vi "Main.vi"() -> ()   [LabVIEW 2020]
doc: "Use this template to build a simple state machine design pattern. Each state executes code and determines which state to transition to."
uses:
  Type Definitions/Data.ctl
  Type Definitions/Error Levels.ctl
  <userlib>/RxnRover/DynamicReentrant/Dynamic Reentrant.lvlib
  <userlib>/RxnRover/DynamicReentrant/src/Type Defs/Message.ctl
  Plugin Servers/Controller Array/Controller Array.lvclass
  Plugin Servers/Controller/Generic Plugin.lvclass
  <vilib>/Utility/error.llb/Error Cluster From Error Code.vi
  Sub VIs/Message Queue/test Message Queue.lvlib
  Sub VIs/Message Queue/Enqueue Message (Single).vi
  <vilib>/ErrorRing/Error Ring.xnode
  Plugin Servers/Controller/Controller Type.ctl
  Plugin Servers/Controller Array/Searchable Properties.ctl
  Plugin Servers/Generic Optimizer/Generic Optimizer.lvclass
  events/Process Stopped Cluster.ctl
  Plugin Servers/Parameter to Hardware Map/Parameter to Hardware Map.lvclass
  Experiment/Experiment Manager/Experiment Manager.lvlib
  Plugin Servers/Controller/Minimal Controller Cluster.ctl
  Plugin Servers/Parameter to Hardware Map/Minimal Pair Cluster.ctl
  Plugin Servers/Parameter to Hardware Map/Minimal Map.ctl
  Experiment/Experiment File/Experiment File Cluster.ctl
  Experiment/Experiment File/Experiment File.lvlib
  Plugin Manager/Plugin Types.ctl
  Plugin Manager/Plugin Manager.lvlib
  Plugin Manager/Plugin Details.ctl
panel:
  in  "Stop Hardware Run Btn":bool
  in  "Start Hardware Run Btn":bool
  in  "Exit":bool
  in  "Stop Analyzer Btn":bool
  in  "Load Analyzer Btn":bool
  in  "Stop Optimizer Btn":bool
  in  "Load Optimizer Btn":bool
  in  "Stop Controller Btn":bool
  in  "Load Control Panel":bool
  in  "Auto Param Passing":bool=TRUE
  in  "Reassign Parameters":bool
  in  "Reject Suggestions":bool
  in  "Accept Suggestions":bool
  in  "Select a Plugin":u16(ring) items=["None", "Mock Pump 1", "Mock Pump 2", "Mock Pump 3", "Mock Temperature Controller"]
  out "# of analyzers cached":i32
  out "# of optimizers cached":i32
  out "# of processes cached":i32
  in  "List of Running Plugins":i32(listbox)=-1
  out "Status Bar Text":string
  # "Manual Control"
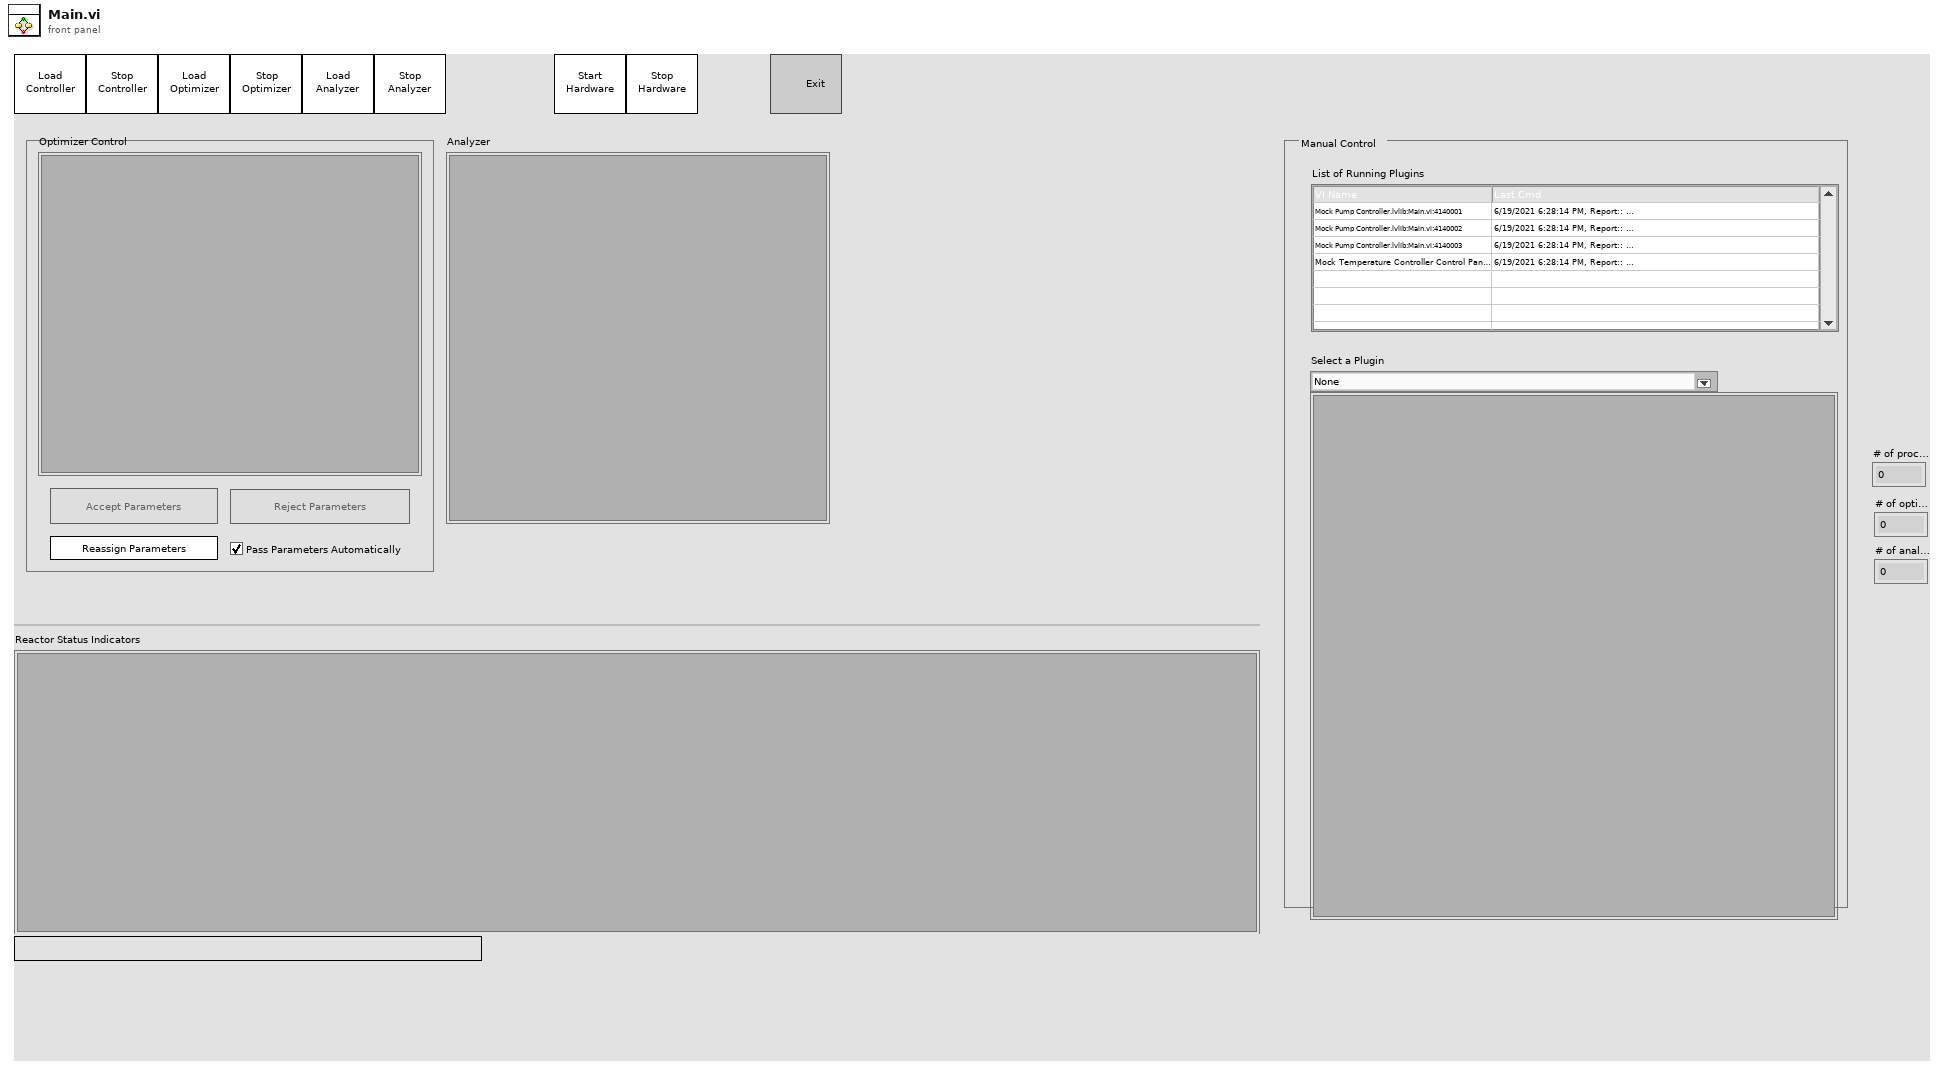
[diagram p1: front panel]
types:
  T1 = enum32{"Invalid", "Standard", "Closed", "Hidden", "Minimized", "Maximized"}
  T2 = typedef "Data.ctl" = cluster{"Main VI Queue":refnum<queue>, "Process Queue References":refnum<queue>[], "Message Queue":refnum<queue>, "Visible Hardware VI":string, "Current Message":T3, "Message History":string[][], "Hardware":cluster{"Process Cache":refnum<class "Controller Array.lvclass">, "Plugins":T4[]}, "Optimizers":cluster{"Process Cache":refnum<class "Controller Array.lvclass">, "Plugins":T4[], "First parameters?":bool, "New Parameters":cluster{"Time Stamp":timestamp, "Names":string[], "Values":dbl[]}}, "Parameter to Hardware Map":refnum<class "Parameter to Hardware Map.lvclass">, "Analyzers":cluster{"Process Cache":refnum<class "Controller Array.lvclass">, "Plugins":T4[]}, "Log Directory":path, "Auto Pass Parameters":bool, "Experiment":cluster{"Name":string, "File Path":path, "File Extension":string, "File Cluster":T7}}
  T3 = typedef "Dynamic Reentrant.lvlib/Message.ctl" = cluster{"Source":string, "Destination":string, "Time Stamp":timestamp, "Command":string, "Data":variant}
  T4 = typedef "Plugin Manager.lvlib/Plugin Details.ctl" = cluster{"Plugin Name":string, "Controller Type":T5, "Control Panel Path":path, "Plugin Type":T6}
  T5 = typedef "Generic Plugin.lvclass/Controller Type.ctl" = enum16{"Invalid", "Temperature Controller", "Pump Controller", "Generic Optimizer", "LC Parser"}
  T6 = typedef "Plugin Manager.lvlib/Plugin Types.ctl" = enum16{"Invalid", "Optimizer", "Analyzer", "Hardware"}
  T7 = typedef "Experiment File.lvlib/Experiment File Cluster.ctl" = cluster{"Hardware List":T8[], "Optimizer List":T8[], "Analyzer List":T8[], "Parameter to Hardware Map":T9}
  T8 = typedef "Generic Plugin.lvclass/Minimal Controller Cluster.ctl" = cluster{"Name":string, "Controller Type":string, "Control Panel Path":string, "Resource":string}
  T9 = typedef "Parameter to Hardware Map.lvclass/Minimal Map.ctl" = T10[]
  T10 = typedef "Parameter to Hardware Map.lvclass/Minimal Pair Cluster.ctl" = cluster{"key":string, "values":T8[]}
  T11 = typedef "Error Levels.ctl" = enum16{"Fatal", "Warning"}
  T12 = typedef "Controller Array.lvclass/Searchable Properties.ctl" = enum16{"Name", "Controller Type"}
  T13 = cluster{"Time Stamp":timestamp, "Names":string[], "Values":dbl[]}
  T14 = enum8{"Enabled", "Disabled", "Disabled and Grayed Out"}
  T15 = typedef "Parameter to Hardware Map.lvclass/Pair.ctl" = cluster{"key":string, "values":refnum<class "Generic Plugin.lvclass">[]}
  T16 = typedef "Process Stopped Cluster.ctl" = cluster{"Name":string, "Type":enum16{"Hardware", "Optimizer", "Analyzer"}}
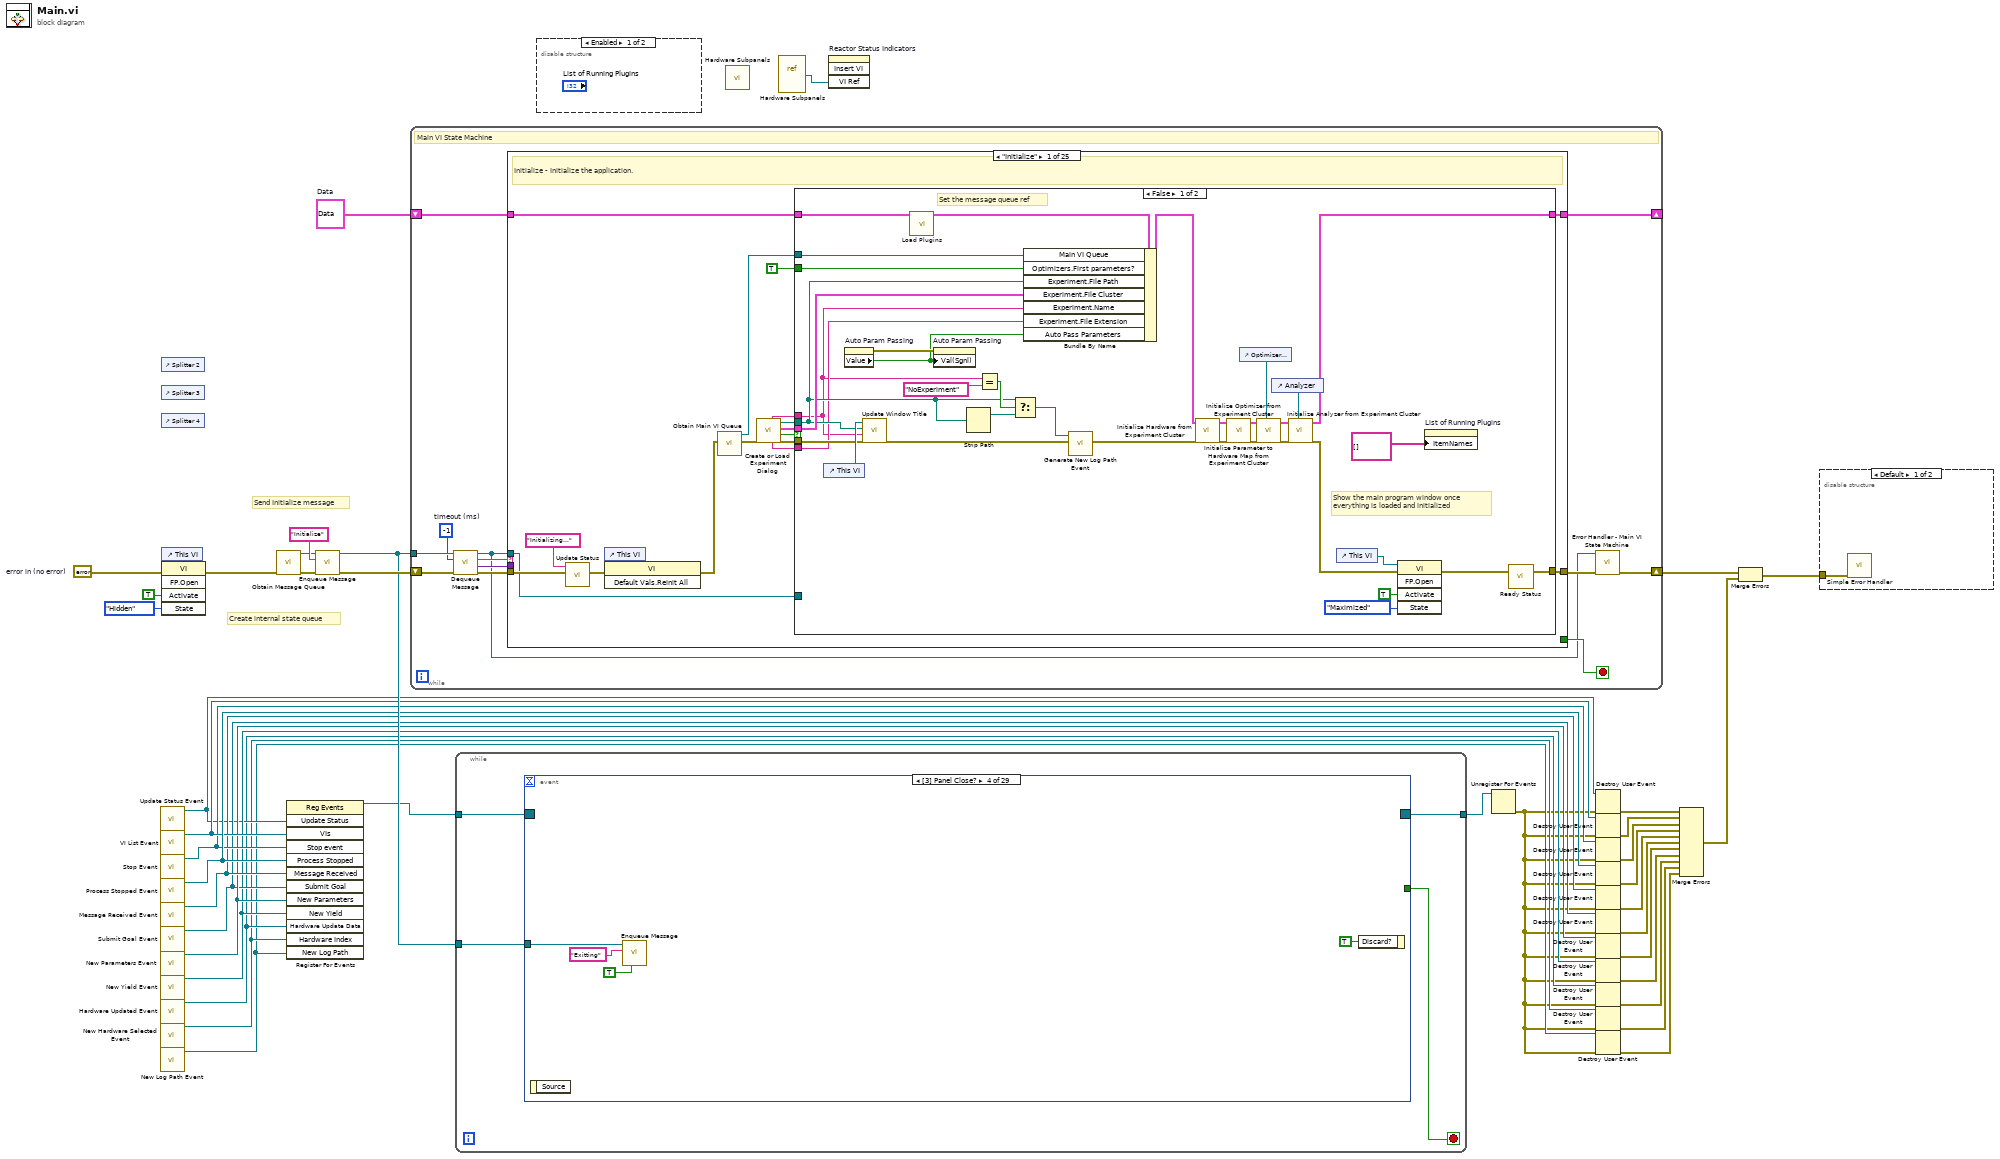
[diagram p0: block diagram]
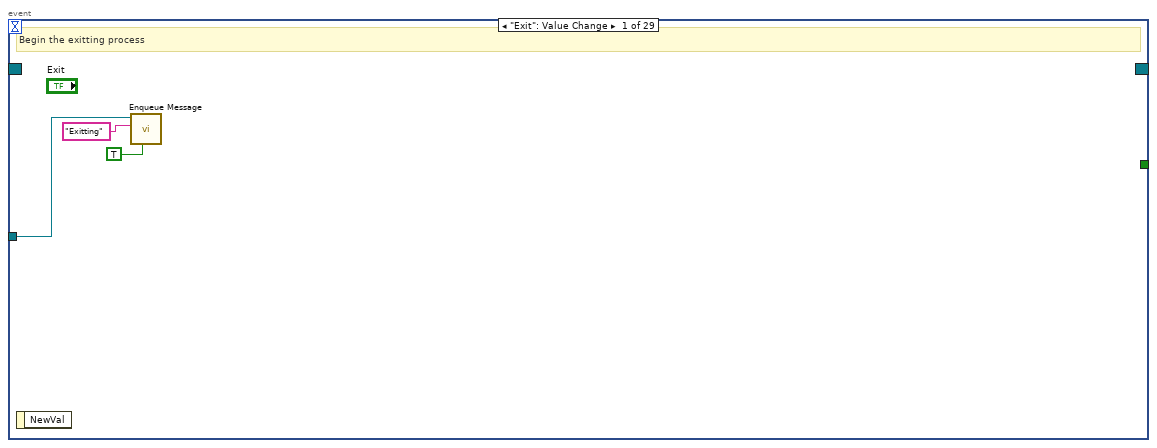
[diagram p2: hidden frame]
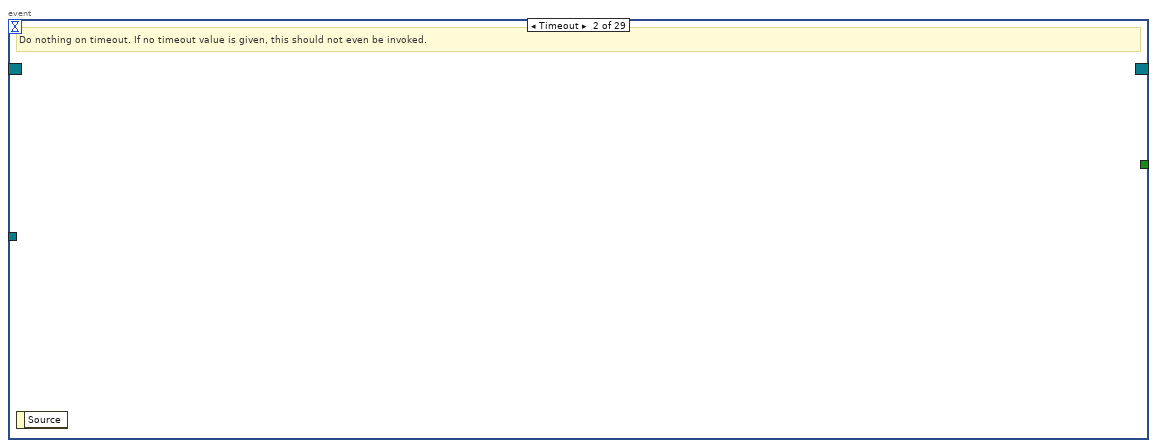
[diagram p3: hidden frame]
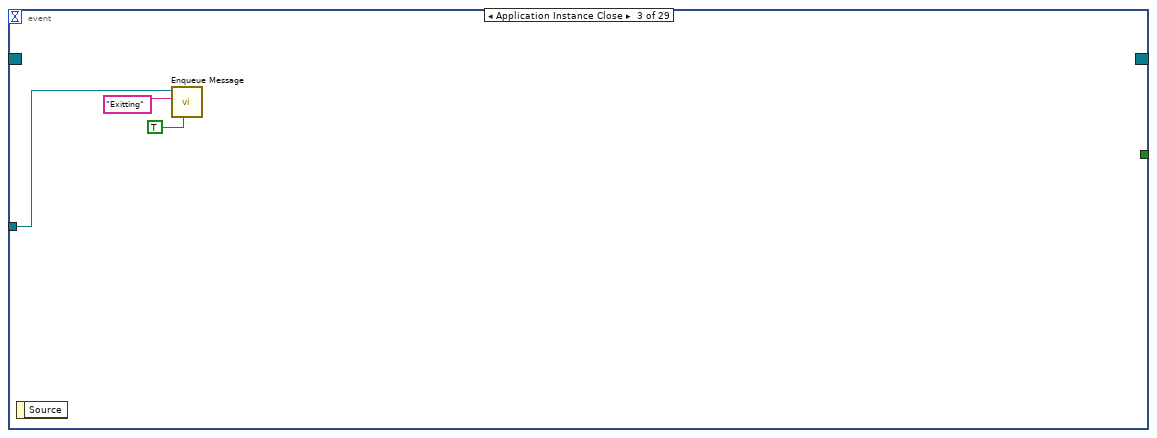
[diagram p4: hidden frame]
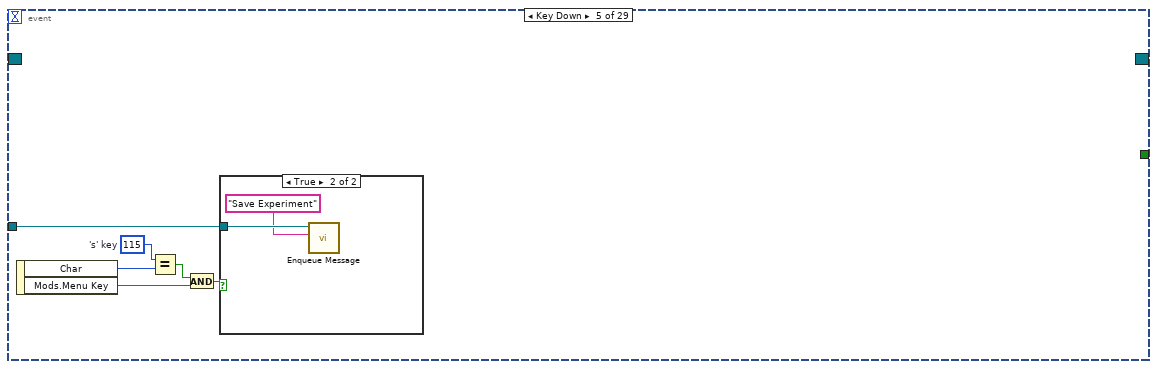
[diagram p5: hidden frame]
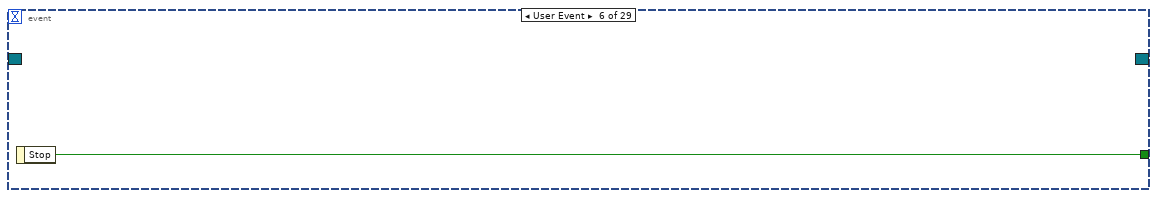
[diagram p7: hidden frame]
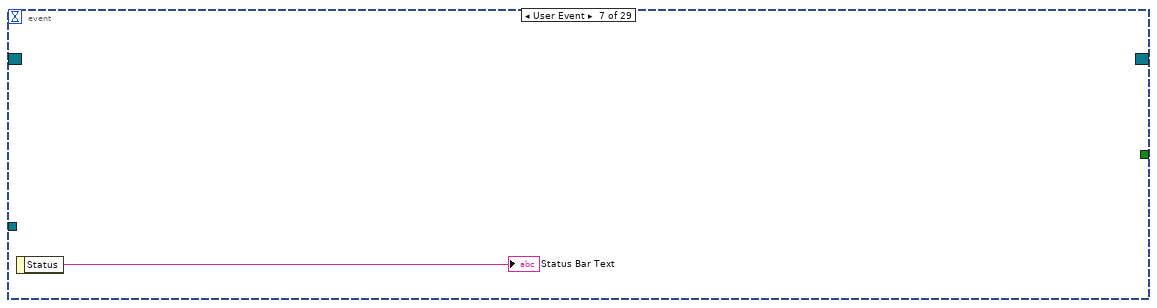
[diagram p8: hidden frame]
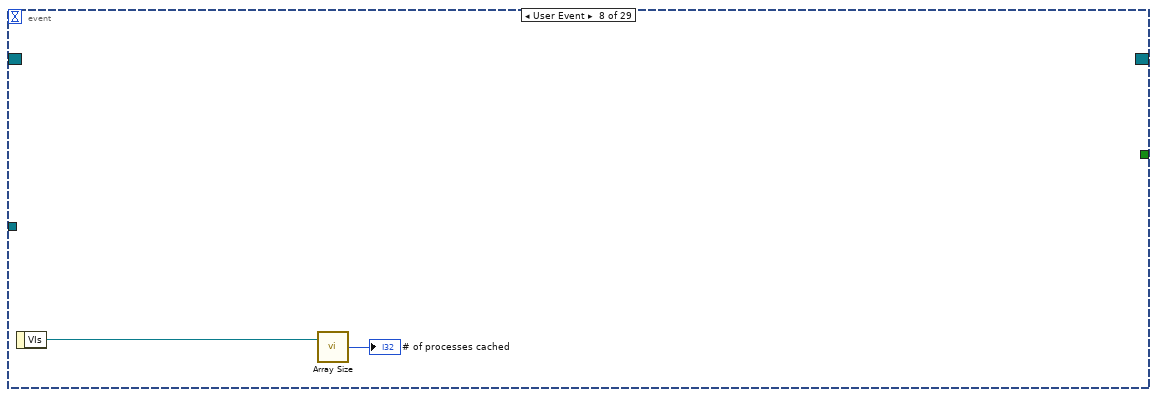
[diagram p9: hidden frame]
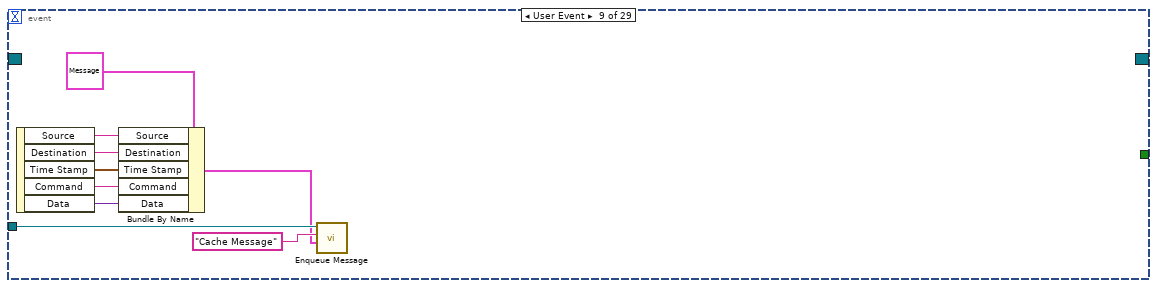
[diagram p10: hidden frame]
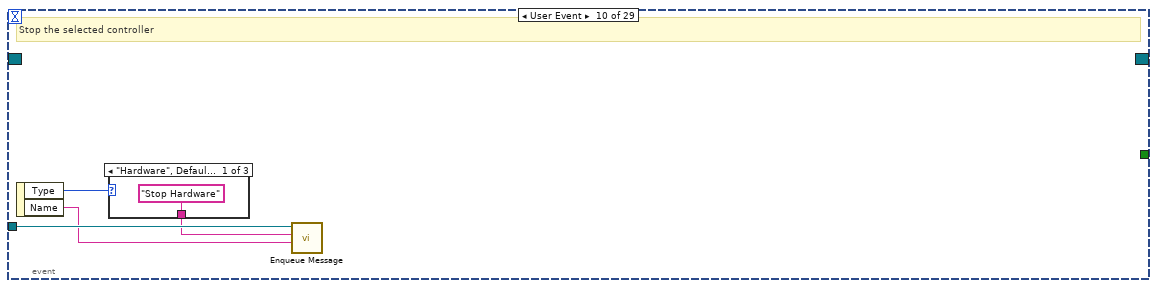
[diagram p11: hidden frame]
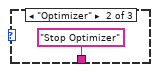
[diagram p12: hidden frame]
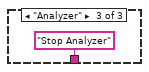
[diagram p13: hidden frame]
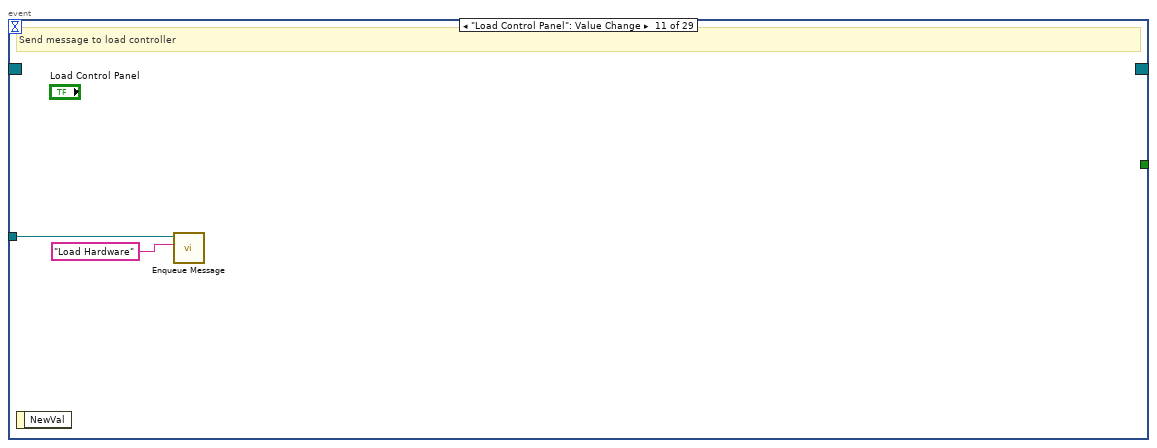
[diagram p14: hidden frame]
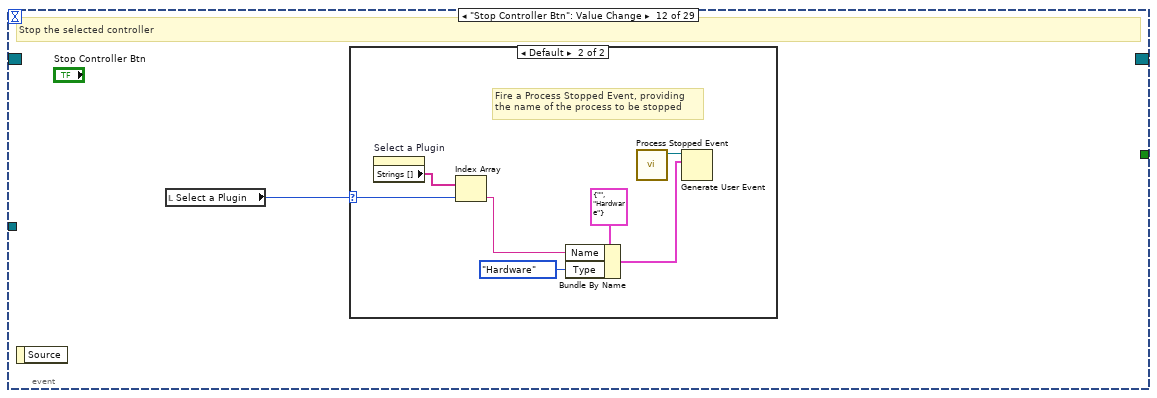
[diagram p15: hidden frame]
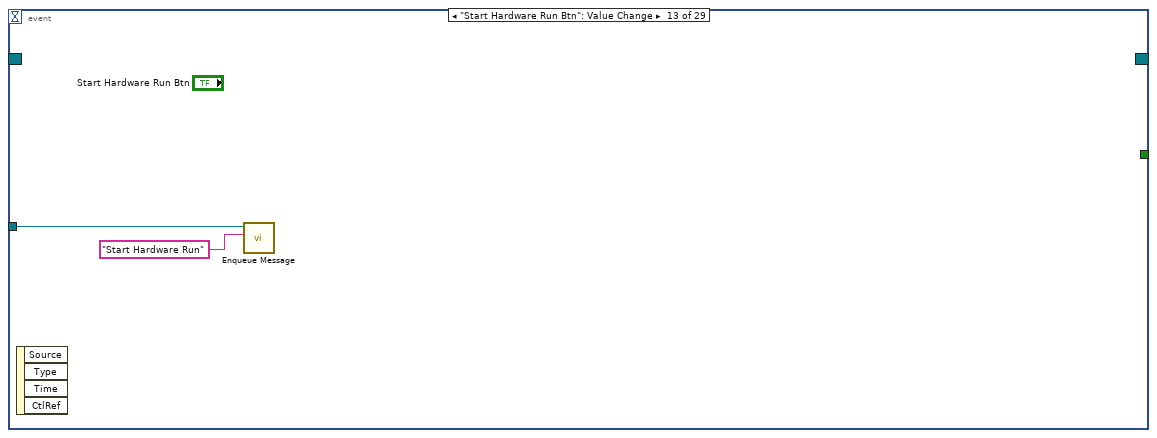
[diagram p17: hidden frame]
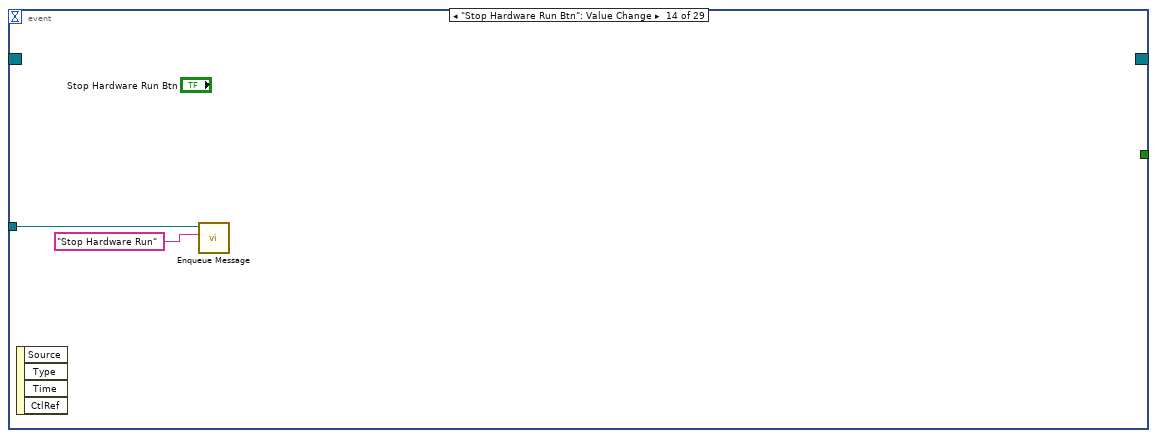
[diagram p18: hidden frame]
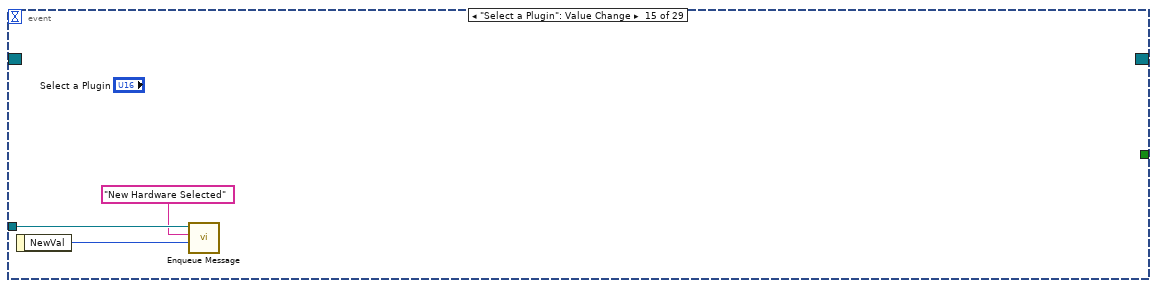
[diagram p19: hidden frame]
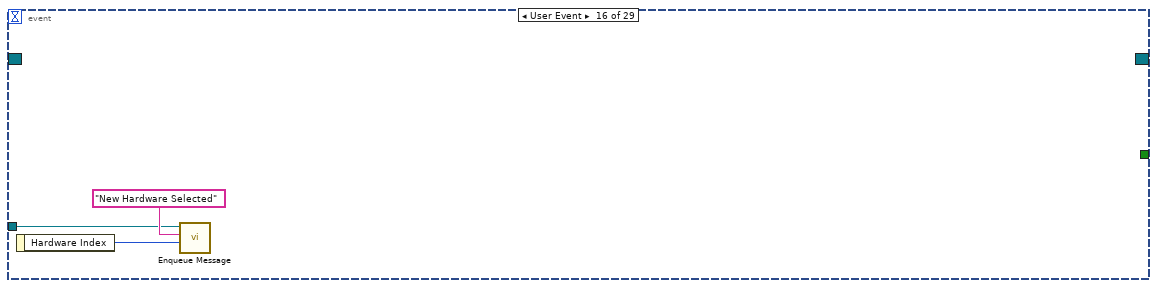
[diagram p20: hidden frame]
diagram:
  w14 = errorcluster {"status"=FALSE, "code"=0, "source"=""}  # error in (no error)
  w26 = T2 {"Main VI Queue"=refnum, "Process Queue References"=[], "Message Queue"=refnum, "Visible Hardware VI"="", "Current Message"={"Source"="", "Destination"="", "Time Stamp"=timestamp(0 s since 1904-01-01), "Command"="", "Data"=variant(string "")}, "Message History"=[], "Hardware"={"Process Cache"=refnum, "Plugins"=[{"Plugin Name"="", "Controller Type"=enum."Invalid", "Control Panel Path"=path "", "Plugin Type"=enum."Optimizer"}, {"Plugin Name"="", "Controller Type"=enum."Invalid", "Control Panel Path"=path "", "Plugin Type"=enum."Optimizer"}, {"Plugin Name"="", "Controller Type"=enum."Invalid", "Control Panel Path"=path "", "Plugin Type"=enum."Optimizer"}, {"Plugin Name"="", "Controller Type"=enum."Invalid", "Control Panel Path"=path "", "Plugin Type"=enum."Optimizer"}]}, "Optimizers"={"Process Cache"=refnum, "Plugins"=[{"Plugin Name"="Deep Reaction Optimizer", "Controller Type"=enum."Invalid", "Control Panel Path"=path "", "Plugin Type"=enum."Optimizer"}, {"Plugin Name"="..\\Optimizers\\Deep Reaction Optimizer\\Control Panel\\Main.vi", "Controller Type"=enum."Invalid", "Control Panel Path"=path "", "Plugin Type"=enum."Optimizer"}, {"Plugin Name"="..\\Optimizers\\Deep Reaction Optimizer\\Source - zmq\\start_inference.bat", "Controller Type"=enum."Invalid", "Control Panel Path"=path "", "Plugin Type"=enum."Optimizer"}], "First parameters?"=FALSE, "New Parameters"={"Time Stamp"=timestamp(0 s since 1904-01-01), "Names"=[], "Values"=[]}}, "Parameter to Hardware Map"=refnum, "Analyzers"={"Process Cache"=refnum, "Plugins"=[{"Plugin Name"="ChromTech Pump Controller", "Controller Type"=enum."Invalid", "Control Panel Path"=path "", "Plugin Type"=enum."Optimizer"}, {"Plugin Name"="Pump Controller", "Controller Type"=enum."Invalid", "Control Panel Path"=path "", "Plugin Type"=enum."Optimizer"}, {"Plugin Name"="..\\Instrumentation\\ChromTech MX-Class\\Control Panel\\Main.vi", "Controller Type"=enum."Invalid", "Control Panel Path"=path "", "Plugin Type"=enum."Optimizer"}, {"Plugin Name"="", "Controller Type"=enum."Invalid", "Control Panel Path"=path "", "Plugin Type"=enum."Optimizer"}]}, "Log Directory"=path "", "Auto Pass Parameters"=FALSE, "Experiment"={"Name"="", "File Path"=path "", "File Extension"="", "File Cluster"={"Hardware List"=[], "Optimizer List"=[], "Analyzer List"=[], "Parameter to Hardware Map"=[]}}}  # Data
  # "Send Initialize message"
  # "Create internal state queue"
  n1 = call "Update Status Event.vi"() -> ("Update Status"=w8:refnum<user-event>)  [unwired: 11 in]
  n2 = call "VI List Event.vi"() -> ("VIs"=w31:refnum<user-event>)  [unwired: 11 in]
  n3 = call "Stop Event.vi"() -> ("Stop event"=w25:refnum<user-event>)  [unwired: 11 out]
  n4 = call "Process Stopped Event.vi"() -> ("Process Stopped"=w32:refnum<user-event>)  [unwired: 11 in]
  n5 = call "Message Received Event.vi"() -> ("Message Received"=w23:refnum<user-event>)  [unwired: 11 in]
  n6 = call "Submit Goal Event.vi"() -> ("Submit Goal"=w21:refnum<user-event>)  [unwired: 11 in]
  n7 = call "New Parameters Event.vi"() -> ("New Parameters"=w22:refnum<user-event>)  [unwired: 11 in]
  n8 = call "New Yield Event.vi"() -> ("New Yield"=w17:refnum<user-event>)  [unwired: 11 in]
  n9 = call "Hardware Updated Event.vi"() -> ("Hardware Update Data"=w7:refnum<user-event>)  [unwired: 11 in]
  n10 = call "New Hardware Selected Event.vi"() -> ("Hardware Index"=w6:refnum<user-event>)  [unwired: 11 in]
  n11 = call "New Log Path Event.vi"() -> ("New Log Path"=w5:refnum<user-event>)  [unwired: 11 in]
  n12 = control-ref of="Splitter 2"() -> ()  [unwired: 1 out]
  n13 = control-ref of="Splitter 3"() -> ()  [unwired: 1 out]
  n14 = control-ref of="Splitter 4"() -> ()  [unwired: 1 out]
  n15 = control-ref of="This VI"() -> (w12:refnum<vi>)
  n16 = invoke class="VI" method="FP.Open"(reference=w12, error in=w14, "Activate"=TRUE ("Activate?"), "State"=T1."Hidden") -> (error out=w13:errorcluster)  [unwired: 1 in, 4 out]
  n17 = call "Obtain Message Queue.vi"("error in (no error)"=w13) -> ("error out"=w38:errorcluster, "Message Queue"=w35:refnum<queue>)  [unwired: 9 in]
  n18 = register-events(w8, w31, w25, w32, w23, w21, w22, w17, w7, w6, w5) -> (reference out=w33:refnum<event-registration>)  [unwired: 2 in, 1 out]
  n19 = call-poly "Enqueue Message.vi"("error in (no error)"=w38, "Message"="Initialize", "Message Queue"=w35) -> ("error out"=w37:errorcluster, "dup Message Queue"=w34:refnum<queue>)  [unwired: 7 in]
  n20 = while {
    shift-right: [w52] -> _
    shift-left: w26 -> [w49]
    shift-right: [w42] -> w40
    shift-left: w37 -> [w51]
    tunnel: w34 -> [w47]
    stop <- w50 stop-if-true
    w44 = -1  # timeout (ms)
    # "Main VI State Machine"
    n21 = call "Dequeue Message.vi"("error in (no error)"=w51, "timeout in ms (-1)"=w44, "Message Queue"=w47) -> ("error out"=w48:errorcluster, "Message Data"=w45:variant, "Message"=w46:string, "dup Message Queue"=w41:refnum<queue>)  [unwired: 5 in]
    n22 = case shown="\"Initialize\"" w46 {
      selector: w46 -> [_ _ _ _ _ _ w246 _ _ _ _ _ _ _ _ _ _ _ _ _ _ _ _ _ _]
      tunnel: [_ _ w138 w175 w236 _ _ _ _ _ _ _ _ _ _ _ _ _ _ _ _ _ _ _ _] -> w50
      tunnel: w49 -> [w68 w119 w136 w143 w232 w244 w248 w257 w274 w295 w327 w374 w400 w417 w429 w447 w504 w530 w577 w598 w603 w627 w655 w680 w737]
      tunnel: [w56 w119 w136 w167 w225 w245 w248 w257 w272 w284 w331 w374 w400 w417 w429 w437 w505 w516 w566 w596 w603 w627 w655 w670 w738] -> w52
      tunnel: w48 -> [w69 w115 w131 w168 w235 w241 _ w258 w278 w297 w339 w375 w391 w414 w426 w444 w511 w528 w576 w597 w606 w635 w657 w677 w744]
      tunnel: [w63 w118 w131 w174 w231 w240 w247 w256 w277 w293 w340 w373 w390 w418 w430 w441 w510 w531 w578 w595 w599 w625 w652 w674 w743] -> w43
      tunnel: w41 -> [w55 w113 _ w173 _ _ _ _ _ _ _ _ _ _ _ _ _ w519 w567 _ _ _ w651 _ _]
      tunnel: w45 -> [_ _ _ _ _ w242 _ _ w276 _ w336 w376 _ _ _ _ w509 w523 _ w594 w604 _ _ _ w742]
      frame "Initialize" {
        # "Initialize - Initialize the application."
        n23 = call "Update Status.vi"("error in (no error)"=w69, "Status Bar Text"="Initializing...") -> ("error out"=w66:errorcluster)  [unwired: 9 in]
        n24 = control-ref of="This VI"() -> (w70:refnum<vi>)
        n25 = invoke class="VI" method="Default Vals.Reinit All"(reference=w70, error in=w66) -> (error out=w58:errorcluster)  [unwired: 1 in, 2 out]
        n26 = call <userlib>:"Obtain Main VI Queue.vi"("error in (no error)"=w58) -> ("error out"=w57:errorcluster, "Main VI Queue"=w67:refnum<queue>)  [unwired: 9 in]
        n27 = call "Create or Load Experiment Dialog.vi"("error in (no error)"=w57) -> ("error out"=w60:errorcluster, "Cancelled?"=w54:bool, "Experimental File Cluster"=w62:T7, "Experiment File Path"=w59:path, "Experiment File Extension"=w53:string, "Experiment Name"=w61:string)  [unwired: 5 in]
        n28 = case shown="False" w54 {
          tunnel: w68 -> [w105 w110]
          tunnel: w67 -> [w103 _]
          tunnel: TRUE ("Optimizers.First parameters?") -> [w102 _]
          tunnel: [w97 errorcluster {"status"=FALSE, "code"=0, "source"=""} ("error out")] -> w63
          tunnel: w62 -> [w96 _]
          tunnel: w61 -> [w72 _]
          tunnel: w60 -> [w94 _]
          tunnel: w59 -> [w75 _]
          tunnel: [w88 w110] -> w56
          tunnel: w55 -> [_ w107]
          tunnel: w53 -> [w73 _]
          frame False {
            # "Show the main program window once\neverything is loaded and initialized"
            # "Set the message queue ref"
            n29 = control-ref of="This VI"() -> (w95:refnum<vi>)
            n30 = property on="Auto Param Passing" class="Bool (strict)"() -> (error out=w80:errorcluster, "Value"=w78:bool)  [unwired: 2 in, 1 out]
            n31 = call "Update Window Title.vi"("error in (no error)"=w94, "Experiment Name"=w72, "Experiment File Path"=w75, "VI in"=w95) -> ("error out"=w93:errorcluster)  [unwired: 7 in]
            n32 = call "Load Plugins.vi"("Data in"=w105) -> ("Data out"=w81:T2)  [unwired: 9 in, 1 out]
            n33 = property on="Auto Param Passing" class="Bool (strict)"(error in=w80, "Val(Sgnl)"=w78) -> ()  [unwired: 1 in, 2 out]
            n34 = Strip Path(path=w75) -> (stripped path=w76:path)  [unwired: 1 out]
            n35 = Equal?(x=w72, y="NoExperiment") -> (x = y?=w77:bool)
            n36 = Select(t=w75, s=w77, f=w76) -> (s? t:f=w74:path)
            n37 = Bundle By Name(cluster=w81, "Main VI Queue"=w103, "Optimizers.First parameters?"=w102, "Experiment.File Path"=w75, "Experiment.File Cluster"=w96, "Experiment.Name"=w72, "Experiment.File Extension"=w73, "Auto Pass Parameters"=w78) -> (w92:T2)
            n38 = call "Generate New Log Path Event.vi"("error in (no error)"=w93, "New Log Path"=w74) -> ("error out"=w79:errorcluster)  [unwired: 9 in]
            n39 = call "Initialize Hardware from Experiment Cluster.vi"("error in (no error)"=w79, "Reaction Rover Data"=w92) -> ("error out"=w87:errorcluster, "Reaction Rover Data out"=w85:T2)  [unwired: 7 in, 1 out]
            n40 = call "Initialize Parameter to Hardware Map from Experiment Cluster.vi"("error in (no error)"=w87, "Reaction Rover Data in"=w85) -> ("error out"=w86:errorcluster, "Reaction Rover Data out"=w84:T2)  [unwired: 8 in]
            n41 = control-ref of="Optimizer Control"() -> (w83:refnum<vi>)
            n42 = call "Initialize Optimizer from Experiment Cluster.vi"("Optimizer Control"=w83, "error in (no error)"=w86, "Reaction Rover Data"=w84) -> ("error out"=w91:errorcluster, "Reaction Rover Data out"=w89:T2)  [unwired: 6 in, 1 out]
            n43 = control-ref of="Analyzer"() -> (w82:refnum<vi>)
            n44 = call "Initialize Analyzer from Experiment Cluster.vi"("Analyzer Panel"=w82, "error in (no error)"=w91, "Reaction Rover Data"=w89) -> ("error out"=w90:errorcluster, "Reaction Rover Data out"=w88:T2)  [unwired: 6 in, 1 out]
            n45 = control-ref of="This VI"() -> (w100:refnum<vi>)
            n46 = invoke class="VI" method="FP.Open"(reference=w100, error in=w90, "Activate"=TRUE ("Activate?"), "State"=T1."Maximized") -> (error out=w101:errorcluster)  [unwired: 1 in, 4 out]
            n47 = property on="List of Running Plugins" class="MCListbox (strict)"("ItemNames"=string[][] [] ("Item Names")) -> ()  [unwired: 2 in, 2 out]
            n48 = call "Ready Status.vi"("error in (no error)"=w101) -> ("error out"=w97:errorcluster)  [unwired: 2 in]
          }
          frame True {
            n49 = call-poly "Enqueue Message.vi"("Priority Message? (F)"=TRUE, "Message"="Exit", "Message Queue"=w107) -> ()  [unwired: 7 in, 2 out]
          }
        }
      }
      frame "Error" {
        # "Handle errors and warnings, determining if the error warrants program shutdown."
        n50 = call "Update Status.vi"("error in (no error)"=w115, "Status Bar Text"="Error!") -> ("error out"=w112:errorcluster)  [unwired: 9 in]
        n51 = Unbundle By Name(w112) -> ("code"=w117:i32)
        n52 = Less Than 0?(x=w117) -> (x < 0?=w116:bool)
        n53 = case shown="True" w116 {
          tunnel: [Error_Levels."Warning" Error_Levels."Fatal"] -> w114
          frame False {
          }
          frame True {
          }
        }
        n54 = case shown="\"Fatal\", Default" w114 {
          tunnel: [w123 w126] -> w118
          tunnel: w112 -> [w124 w128]
          tunnel: w113 -> [w122 _]
          frame "Fatal", Default {
            n55 = call <vilib>:"Simple Error Handler.vi"("error in (no error)"=w124) -> ("error out"=w125:errorcluster)  [unwired: 4 in, 4 out]
            n56 = call <vilib>:"Clear Errors.vi"("error in (no error)"=w125) -> ("error out"=w120:errorcluster)  [unwired: 5 in, 1 out]
            n57 = call-poly "Enqueue Message.vi"("error in (no error)"=w120, "Message"="Exitting", "Message Queue"=w122) -> ("error out"=w123:errorcluster)  [unwired: 7 in, 1 out]
          }
          frame "Warning" {
            n58 = call <vilib>:"Simple Error Handler.vi"("error in (no error)"=w128) -> ("error out"=w127:errorcluster)  [unwired: 4 in, 4 out]
            n59 = call <vilib>:"Clear Errors.vi"("error in (no error)"=w127) -> ("error out"=w126:errorcluster)  [unwired: 5 in, 1 out]
          }
        }
      }
      frame "Exit" {
        w132 = TRUE  # Stop
        w138 = TRUE  # Stop Loop?
        # "Release these queue references in a delayed way. We do not want to release them before the process VI has received the message."
        # "Exit - Exit the application."
        n60 = call "Stop Event.vi"() -> ("Stop event"=w134:refnum<user-event>)  [unwired: 11 out]
        n61 = Generate User Event(user event=w134, event data cluster=w132) -> (error out=w133:errorcluster)  [unwired: 2 in, 1 out]
        n62 = call <vilib>:"Simple Error Handler.vi"("error in (no error)"=w133) -> ()  [unwired: 4 in, 5 out]
        n63 = Unbundle By Name(w136) -> ("Process Queue References"=w137:refnum<queue>[], "Main VI Queue"=w135:refnum<queue>)
        n64 = for {
          tunnel: w137 -> [w139] mode=indexing
          n65 = Release Queue(queue=w139) -> ()  [unwired: 2 in, 3 out]
        }
        n66 = Release Queue(queue=w135) -> ()  [unwired: 2 in, 3 out]
      }
      frame "Exitting" {
        w174 = errorcluster {"status"=FALSE, "code"=0, "source"=""}  # error out
        w175 = FALSE  # Stop Loop?
        # "Make sure each hardware has been\ninstructed to stop before attempting\nto shut down the controllers"
        # "Send Exit Command to all open Process VIs. Doing a Force Destroy on all the queues of the process VIs will also have the same effect, based on how the process VI is currently written."
        # "Errors need to be shown here or they will be ignored since there is no room to enter the Error state anymore."
        # "Start at the back of the array"
        # "Begin exitting the application"
        n67 = Unbundle By Name(w143) -> ("Optimizers.Process Cache"=w165:refnum<class "Controller Array.lvclass">)
        n68 = call "Update Status.vi"("error in (no error)"=w168, "Status Bar Text"="Exitting") -> ("error out"=w145:errorcluster)  [unwired: 9 in]
        n69 = call "Save Reaction Rover Data to Experiment File.vi"("error in (no error)"=w145, "Reaction Rover Data"=w143) -> ("error out"=w144:errorcluster)  [unwired: 7 in, 2 out]
        n70 = call "Array Size.vi"("Controller Array in"=w165, "error in (no error)"=w144) -> ("Controller Array out"=w160:refnum<class "Controller Array.lvclass">, "size(s)"=w161:i32, "error out"=w162:errorcluster)
        n71 = Decrement(x=w161) -> (x-1=w159:i32)
        n72 = for {
          N: w161 -> [_]
          shift-right: [w195] -> w151
          shift-left: w162 -> [w208]
          tunnel: w159 -> [w203]
          tunnel: w160 -> [w202]
          shift-right: [w194] -> w153
          shift-left: w143 -> [w197]
          i -> [w204]
          n73 = Subtract(x=w203, y=w204) -> (x-y=w205:i32)
          n74 = call "Index Array.vi"("error in (no error)"=w208, "index"=w205, "Controller Array in"=w202) -> ("error out"=w206:errorcluster, "element"=w201:refnum<class "Generic Plugin.lvclass">)  [unwired: 1 out]
          n75 = call "Read Name.vi"("controller in"=w201, "error in (no error)"=w206) -> ("Name"=w199:string, "error out"=w200:errorcluster)  [unwired: 1 out]
          n76 = call "Stop Optimizer VI.vi"("error in (no error)"=w200, "Blocking (T)"=TRUE, "Process Name"=w199, "Data in"=w197) -> ("error out"=w196:errorcluster, "Data out"=w194:T2)  [unwired: 6 in]
          n77 = Unbundle By Name(w194) -> ("Message History"=w198:string[][])
          n78 = invoke on="Optimizer Control" class="SubPnl" method="Remove VI"(error in=w196) -> (error out=w195:errorcluster)  [unwired: 2 in, 2 out]
          n79 = property on="List of Running Plugins" class="MCListbox (strict)"("ItemNames"=w198) -> ()  [unwired: 2 in, 2 out]
        }
        n80 = Unbundle By Name(w153) -> ("Analyzers.Process Cache"=w154:refnum<class "Controller Array.lvclass">)
        n81 = call "Array Size.vi"("Controller Array in"=w154, "error in (no error)"=w151) -> ("Controller Array out"=w157:refnum<class "Controller Array.lvclass">, "size(s)"=w156:i32, "error out"=w155:errorcluster)
        n82 = Decrement(x=w156) -> (x-1=w158:i32)
        n83 = for {
          N: w156 -> [_]
          shift-right: [w180] -> w149
          shift-left: w155 -> [w193]
          tunnel: w158 -> [w188]
          tunnel: w157 -> [w187]
          shift-right: [w179] -> w152
          shift-left: w153 -> [w182]
          i -> [w189]
          n84 = Subtract(x=w188, y=w189) -> (x-y=w190:i32)
          n85 = call "Index Array.vi"("error in (no error)"=w193, "index"=w190, "Controller Array in"=w187) -> ("error out"=w191:errorcluster, "element"=w186:refnum<class "Generic Plugin.lvclass">)  [unwired: 1 out]
          n86 = call "Read Name.vi"("controller in"=w186, "error in (no error)"=w191) -> ("Name"=w184:string, "error out"=w185:errorcluster)  [unwired: 1 out]
          n87 = call "Stop Analyzer VI.vi"("error in (no error)"=w185, "Blocking (T)"=TRUE, "Process Name"=w184, "Data in"=w182) -> ("error out"=w181:errorcluster, "Data out"=w179:T2)  [unwired: 6 in]
          n88 = Unbundle By Name(w179) -> ("Message History"=w183:string[][])
          n89 = invoke on="Analyzer" class="SubPnl" method="Remove VI"(error in=w181) -> (error out=w180:errorcluster)  [unwired: 2 in, 2 out]
          n90 = property on="List of Running Plugins" class="MCListbox (strict)"("ItemNames"=w183) -> ()  [unwired: 2 in, 2 out]
        }
        n91 = Unbundle By Name(w152) -> ("Hardware.Process Cache"=w150:refnum<class "Controller Array.lvclass">)
        n92 = call "Read Array.vi"("error in (no error)"=w149, "Controller Array in"=w150) -> ("error out"=w147:errorcluster, "Array"=w148:refnum<class "Generic Plugin.lvclass">[])  [unwired: 7 in, 1 out]
        n93 = for {
          tunnel: w148 -> [w178] mode=indexing
          shift-right: [w176] -> w146
          shift-left: w147 -> [w177]
          n94 = call "Send Stop Message.vi"("error in (no error)"=w177, "Generic Controller in"=w178) -> ("error out"=w176:errorcluster)  [unwired: 8 in, 1 out]
        }
        n95 = call "Array Size.vi"("Controller Array in"=w150, "error in (no error)"=w146) -> ("Controller Array out"=w164:refnum<class "Controller Array.lvclass">, "size(s)"=w171:i32, "error out"=w163:errorcluster)
        n96 = Decrement(x=w171) -> (x-1=w170:i32)
        n97 = for {
          N: w171 -> [_]
          shift-right: [w211] -> w141
          shift-left: w163 -> [w222]
          tunnel: w170 -> [w218]
          shift-right: [w213] -> w167
          shift-left: w152 -> [w214]
          tunnel: w164 -> [w215]
          i -> [w217]
          n98 = Subtract(x=w218, y=w217) -> (x-y=w216:i32)
          n99 = call "Index Array.vi"("error in (no error)"=w222, "index"=w216, "Controller Array in"=w215) -> ("error out"=w220:errorcluster, "element"=w221:refnum<class "Generic Plugin.lvclass">)  [unwired: 1 out]
          n100 = call "Read Name.vi"("controller in"=w221, "error in (no error)"=w220) -> ("Name"=w210:string, "error out"=w219:errorcluster)  [unwired: 1 out]
          n101 = call "Stop Process VI.vi"("error in (no error)"=w219, "Blocking (T)"=TRUE, "Process Name"=w210, "Data in"=w214) -> ("error out"=w211:errorcluster, "Data out"=w213:T2)  [unwired: 6 in]
          n102 = Unbundle By Name(w213) -> ("Message History"=w212:string[][])
          n103 = property on="List of Running Plugins" class="MCListbox (strict)"("ItemNames"=w212) -> ()  [unwired: 2 in, 2 out]
        }
        n104 = invoke on="Selected Plugin" class="SubPnl" method="Remove VI"(error in=w141) -> (error out=w140:errorcluster)  [unwired: 2 in, 2 out]
        n105 = call <vilib>:"Clear Errors.vi"("error in (no error)"=w140) -> ("error out"=w142:errorcluster)  [unwired: 5 in, 1 out]
        n106 = call-poly "Enqueue Message.vi"("Priority Message? (F)"=TRUE, "error in (no error)"=w142, "Message"="Exit", "Message Queue"=w173) -> ()  [unwired: 6 in, 2 out]
        n107 = call <vilib>:"Simple Error Handler.vi"("error in (no error)"=w140) -> ()  [unwired: 4 in, 5 out]
      }
      frame "Save Experiment" {
        w236 = FALSE  # Stop Loop?
        # "Save the current state to the experiment file."
        n108 = call "Update Status.vi"("error in (no error)"=w235, "Status Bar Text"="Saving...") -> ("error out"=w233:errorcluster)  [unwired: 9 in]
        n109 = call "Save Reaction Rover Data to Experiment File.vi"("error in (no error)"=w233, "Reaction Rover Data"=w232) -> ("error out"=w228:errorcluster, "Reaction Rover Data out"=w225:T2)  [unwired: 7 in, 1 out]
        n110 = Unbundle By Name(w225) -> ("Experiment.File Path"=w224:path, "Experiment.Name"=w223:string)
        n111 = control-ref of="This VI"() -> (w226:refnum<vi>)
        n112 = call "Update Window Title.vi"("error in (no error)"=w228, "Experiment Name"=w223, "Experiment File Path"=w224, "VI in"=w226) -> ("error out"=w227:errorcluster)  [unwired: 7 in]
        n113 = call "Set Unsaved Changes in Title.vi"("VI in"=w226, "error in (no error)"=w227, "Unsaved changes? (F)"=FALSE) -> ("error out"=w230:errorcluster)  [unwired: 8 in]
        n114 = call "Ready Status.vi"("error in (no error)"=w230) -> ("error out"=w231:errorcluster)  [unwired: 2 in]
      }
      frame "Cache Message" {
        # "Always cache the message in the history"
        n115 = Variant To Data(error in=w241, type=T3 {"Source"="", "Destination"="", "Time Stamp"=timestamp(0 s since 1904-01-01), "Command"="", "Data"=variant} ("Message"), Variant=w242) -> (data=w239:T3, error out=w240:errorcluster)
        n116 = Unbundle By Name(w244) -> ("Message History"=w237:string[][])
        n117 = call "Cache Message.vi"("Message"=w239, "Message History In"=w237) -> ("Message History Out"=w238:string[][])  [unwired: 9 in]
        n118 = property on="List of Running Plugins" class="MCListbox (strict)"("ItemNames"=w238) -> ()  [unwired: 2 in, 2 out]
        n119 = Bundle By Name(cluster=w244, "Message History"=w238) -> (w245:T2)
      }
      frame Default {
        n120 = xnode "Error Ring"("parameter 0"=w246) -> ("error out"=w247:errorcluster)
      }
      frame "--- Copy this Frame ---" {
        n121 = call "Ready Status.vi"("error in (no error)"=w258) -> ("error out"=w256:errorcluster)  [unwired: 2 in]
      }
      frame "New Log Path" {
        # "Send the new log directory to all plugins"
        # "Update the logging directory."
        n122 = Variant To Data(error in=w278, type=path "", Variant=w276) -> (data=w273:path, error out=w270:errorcluster)
        n123 = Bundle By Name(cluster=w274, "Log Directory"=w273) -> (w272:T2)
        n124 = Unbundle By Name(w272) -> ("Log Directory"=w268:path, "Optimizers.Process Cache"=w259:refnum<class "Controller Array.lvclass">, "Analyzers.Process Cache"=w260:refnum<class "Controller Array.lvclass">, "Hardware.Process Cache"=w271:refnum<class "Controller Array.lvclass">)
        n125 = call "Read Array.vi"("error in (no error)"=w270, "Controller Array in"=w271) -> ("error out"=w267:errorcluster, "Array"=w261:refnum<class "Generic Plugin.lvclass">[])  [unwired: 7 in, 1 out]
        n126 = call "Read Array.vi"("error in (no error)"=w267, "Controller Array in"=w260) -> ("error out"=w266:errorcluster, "Array"=w262:refnum<class "Generic Plugin.lvclass">[])  [unwired: 7 in, 1 out]
        n127 = call "Read Array.vi"("error in (no error)"=w266, "Controller Array in"=w259) -> ("error out"=w265:errorcluster, "Array"=w263:refnum<class "Generic Plugin.lvclass">[])  [unwired: 7 in, 1 out]
        n128 = Build Array (concatenate)(w261, w262, w263) -> (w264:refnum<class "Generic Plugin.lvclass">[])
        n129 = for {
          tunnel: w265 -> [w282]
          tunnel: w264 -> [w281] mode=indexing
          tunnel: [w280] -> w269
          tunnel: w268 -> [w279]
          n130 = call "Send Log Directory Message.vi"("error in (no error)"=w282, "Log Directory"=w279, "Generic Controller in"=w281) -> ("error out"=w280:errorcluster)  [unwired: 7 in, 1 out]
        }
        n131 = call "Ready Status.vi"("error in (no error)"=w269) -> ("error out"=w277:errorcluster)  [unwired: 2 in]
      }
      frame "Load Hardware" {
        w289 = "Select Hardware" ("Window Title")
        # "Load a selected process."
        n132 = Unbundle By Name(w295) -> ("Log Directory"=w291:path, "Hardware.Process Cache"=w292:refnum<class "Controller Array.lvclass">, "Hardware.Plugins"=w290:T4[])
        n133 = call "Update Status.vi"("error in (no error)"=w297, "Status Bar Text"="Loading Hardware...") -> ("error out"=w294:errorcluster)  [unwired: 9 in]
        n134 = call "Load Plugin Dialog.vi"("Plugin Selection Ring Text"=w289, "Window Title"=w289, "error in (no error)"=w294, "Plugin List"=w290) -> ("error out"=w286:errorcluster, "cancelled"=w288:bool, "Instance Name"=w283:string, "Plugin Selected"=w287:T4)  [unwired: 4 in]
        n135 = case shown="False" w288 {
          tunnel: w295 -> [w314 w325]
          tunnel: [w313 w325] -> w284
          tunnel: w292 -> [w312 _]
          tunnel: [w311 w324] -> w285
          tunnel: w286 -> [w305 w324]
          tunnel: w291 -> [w302 _]
          tunnel: w287 -> [w308 _]
          tunnel: w283 -> [w301 _]
          frame False {
            n136 = Unbundle By Name(w308) -> ("Controller Type"=w304:T5, "Control Panel Path"=w303:path)
            n137 = call "Initialize Plugin.vi"("Instance Name (blank for default)"=w301, "error in (no error)"=w305, "Log Directory"=w302, "Plugin Path in"=w303, "Plugin Type"=w304) -> ("error out"=w298:errorcluster, "Failed?"=w299:bool, "Generic Controller out"=w300:refnum<class "Generic Plugin.lvclass">)  [unwired: 4 in]
            n138 = case shown="True" w299 {
              tunnel: w312 -> [w319 w321]
              tunnel: [w318 w323] -> w307
              tunnel: [w317 w321] -> w306
              tunnel: w300 -> [w316 _]
              tunnel: w298 -> [w315 w320]
              frame False {
                n139 = call "Add Hardware.vi"("error in (no error)"=w315, "new plugin"=w316, "Plugin Array in"=w319) -> ("error out"=w318:errorcluster, "Plugin Array out"=w317:refnum<class "Controller Array.lvclass">)  [unwired: 7 in]
              }
              frame True {
                # "Clear \"VI already\nclosed\" error that\nsometimes occurs\non abort"
                n140 = call <vilib>:"Clear Errors.vi"("error in (no error)"=w320, "specific error code to clear (0: all)"=1026) -> ("error out"=w323:errorcluster)  [unwired: 4 in, 1 out]
              }
            }
            n141 = Bundle By Name(cluster=w314, "Hardware.Process Cache"=w306) -> (w313:T2)
            n142 = control-ref of="This VI"() -> (w310:refnum<vi>)
            n143 = call "Set Unsaved Changes in Title.vi"("VI in"=w310, "error in (no error)"=w307, "Unsaved changes? (F)"=TRUE) -> ("error out"=w311:errorcluster)  [unwired: 8 in]
          }
          frame True {
          }
        }
        n144 = call "Ready Status.vi"("error in (no error)"=w285) -> ("error out"=w293:errorcluster)  [unwired: 2 in]
      }
      frame "Stop Hardware" {
        w335 = "Closing hardware" ("Status Bar Text")
        # "Stop the selected process"
        n145 = Variant To Data(error in=w339, type=w335, Variant=w336) -> (data=w334:string, error out=w338:errorcluster)
        n146 = call "Update Status.vi"("Status Bar Text"=w335) -> ("error out"=w337:errorcluster)  [unwired: 10 in]
        n147 = Merge Errors(w337, w338) -> (w333:errorcluster)
        n148 = Unbundle By Name(w327) -> ("Hardware.Process Cache"=w330:refnum<class "Controller Array.lvclass">)
        n149 = call "Search Array.vi"("error in (no error)"=w333, "Search Value"=w334, "Controller Array in"=w330) -> ("error out"=w328:errorcluster, "Controller found"=w329:refnum<class "Generic Plugin.lvclass">, "Index of found"=w326:i32)  [unwired: 1 in, 1 out]
        n150 = case shown="Default" w326 {
          selector: w326 -> [_ w344]
          tunnel: w334 -> [_ w363]
          tunnel: [w341 w361] -> w332
          tunnel: [w342 w358] -> w331
          tunnel: w329 -> [_ w345]
          tunnel: w328 -> [w341 w355]
          tunnel: w327 -> [w342 w346]
          frame -1 {
            # "Do nothing if the plugin was not found"
          }
          frame Default {
            # "Check if it is the last element.\nIf so, the index may remain the\nsame. This also handles when\nthe last hardware is removed, as\nthe \"None\" option (index 0) will be\nselected.\n\nIf it is not the last element in the \nhardware list, then the hardware \nplugin after it is selected."
            # "Stop the hardware before trying\nto shut down the controller"
            n151 = call "Send Stop Message.vi"("error in (no error)"=w355, "Generic Controller in"=w345) -> ("error out"=w354:errorcluster)  [unwired: 8 in, 1 out]
            n152 = call "Stop Process VI.vi"("error in (no error)"=w354, "Blocking (T)"=TRUE, "Process Name"=w363, "Data in"=w346) -> ("error out"=w353:errorcluster, "Data out"=w358:T2)  [unwired: 6 in]
            n153 = Unbundle By Name(w358) -> ("Hardware.Process Cache"=w350:refnum<class "Controller Array.lvclass">)
            n154 = call "Hardware List Updated.vi"("error in (no error)"=w353) -> ("error out"=w351:errorcluster)  [unwired: 10 in]
            n155 = Unbundle By Name(w358) -> ("Message History"=w357:string[][])
            n156 = call "Array Size.vi"("Controller Array in"=w350, "error in (no error)"=w351) -> ("size(s)"=w349:i32, "error out"=w347:errorcluster)  [unwired: 1 out]
            n157 = property on="List of Running Plugins" class="MCListbox (strict)"("ItemNames"=w357) -> ()  [unwired: 2 in, 2 out]
            n158 = Equal?(x=w344, y=w349) -> (x = y?=w348:bool)
            n159 = Increment(x=w344) -> (x+1=w343:i32)
            n160 = Select(t=w344, s=w348, f=w343) -> (s? t:f=w352:i32)
            n161 = call "New Hardware Selected.vi"("error in (no error)"=w347, "Hardware Index"=w352) -> ("error out"=w359:errorcluster)  [unwired: 9 in]
            n162 = control-ref of="This VI"() -> (w362:refnum<vi>)
            n163 = call "Set Unsaved Changes in Title.vi"("VI in"=w362, "error in (no error)"=w359, "Unsaved changes? (F)"=TRUE) -> ("error out"=w361:errorcluster)  [unwired: 8 in]
          }
        }
        n164 = call "Ready Status.vi"("error in (no error)"=w332) -> ("error out"=w340:errorcluster)  [unwired: 2 in]
      }
      frame "New Hardware Selected" {
        # "Update the currently visible hardware control panel"
        n165 = Variant To Data(error in=w375, type=u16 0, Variant=w376) -> (data=w364:u16, error out=w372:errorcluster)
        n166 = Unbundle By Name(w374) -> ("Hardware.Process Cache"=w366:refnum<class "Controller Array.lvclass">)
        n167 = Less Or Equal To 0?(x=w364) -> (x <= 0?=w367:bool)
        n168 = call "Array Size.vi"("Controller Array in"=w366, "error in (no error)"=w372) -> ("size(s)"=w368:i32, "error out"=w371:errorcluster)  [unwired: 1 out]
        n169 = Greater?(x=w364, y=w368) -> (0:w369:bool)
        n170 = Or(x=w367, y=w369) -> (x .or. y?=w370:bool)
        n171 = case shown="False" w370 {
          tunnel: w371 -> [w386 w389]
          tunnel: [w383 w388] -> w373
          tunnel: w364 -> [w381 _]
          tunnel: w366 -> [w380 _]
          tunnel: [w379 w387] -> w365
          tunnel: w364 -> [w379 _]
          frame False {
            # "Load the new plugin front panel."
            n172 = Decrement(x=w381) -> (x-1=w382:u16)
            n173 = call "Index Array.vi"("error in (no error)"=w386, "index"=w382, "Controller Array in"=w380) -> ("error out"=w385:errorcluster, "element"=w384:refnum<class "Generic Plugin.lvclass">)  [unwired: 1 out]
            n174 = control-ref of="Selected Plugin"() -> (w378:refnum<vi>)
            n175 = call "Load Plugin Front Panel.vi"("error in (no error)"=w385, "Sub Panel"=w378, "Generic Controller in"=w384) -> ("error out"=w383:errorcluster)  [unwired: 8 in]
          }
          frame True {
            w387 = u16 0 items=["None", "Mock Pump Controller.lvlib:Main.vi:4140003"] ("Select a Plugin")
            # "Remove any VI present since either \"None\" or an invalid index was given, which could be negative or higher than the max index."
            n176 = invoke on="Selected Plugin" class="SubPnl" method="Remove VI"(error in=w389) -> (error out=w388:errorcluster)  [unwired: 2 in, 2 out]
          }
        }
        n177 = local write "Select a Plugin"(w365) -> ()
      }
      frame "Refresh Hardware Selector" {
        # "Loop over all hardware processes and get their names"
        # "Refreshes the list of harware the user can select for manual control."
        n178 = Unbundle By Name(w400) -> ("Hardware.Process Cache"=w399:refnum<class "Controller Array.lvclass">)
        n179 = call "Array Size.vi"("Controller Array in"=w399, "error in (no error)"=w391) -> ("Controller Array out"=w398:refnum<class "Controller Array.lvclass">, "size(s)"=w396:i32, "error out"=w397:errorcluster)
        n180 = for {
          N: w396 -> [_]
          tunnel: w398 -> [w409]
          shift-right: [w405] -> w392
          shift-left: w397 -> [w407]
          shift-right: [w403] -> w393
          shift-left: string[] ["None"] -> [w404]
          i -> [w408]
          n181 = call "Index Array.vi"("error in (no error)"=w407, "index"=w408, "Controller Array in"=w409) -> ("error out"=w406:errorcluster, "element"=w401:refnum<class "Generic Plugin.lvclass">)  [unwired: 1 out]
          n182 = call "Read Name.vi"("controller in"=w401, "error in (no error)"=w406) -> ("Name"=w402:string, "error out"=w405:errorcluster)  [unwired: 1 out]
          n183 = Build Array (concatenate)(w404, w402) -> (w403:string[])
        }
        n184 = control-ref of="Select a Plugin"() -> (w394:refnum<vi>)
        n185 = property class="Ring (strict)"(reference=w394, error in=w392, "Strings []"=w393) -> (error out=w390:errorcluster)  [unwired: 1 out]
      }
      frame "Start Hardware Run" {
        n186 = Unbundle By Name(w417) -> ("Hardware.Process Cache"=w416:refnum<class "Controller Array.lvclass">)
        n187 = call "Update Status.vi"("error in (no error)"=w414, "Status Bar Text"="Starting hardware run.") -> ("error out"=w411:errorcluster)  [unwired: 9 in]
        n188 = call "Read Array.vi"("error in (no error)"=w411, "Controller Array in"=w416) -> ("error out"=w413:errorcluster, "Array"=w415:refnum<class "Generic Plugin.lvclass">[])  [unwired: 7 in, 1 out]
        n189 = for {
          tunnel: w415 -> [w420] mode=indexing
          shift-right: [w419] -> w412
          shift-left: w413 -> [w421]
          n190 = call "Send Start Message.vi"("error in (no error)"=w421, "Generic Controller in"=w420) -> ("error out"=w419:errorcluster)  [unwired: 8 in, 1 out]
        }
        n191 = call "Ready Status.vi"("error in (no error)"=w412) -> ("error out"=w418:errorcluster)  [unwired: 2 in]
      }
      frame "Stop Hardware Run" {
        n192 = Unbundle By Name(w429) -> ("Hardware.Process Cache"=w428:refnum<class "Controller Array.lvclass">)
        n193 = call "Update Status.vi"("error in (no error)"=w426, "Status Bar Text"="Stopping hardware run.") -> ("error out"=w423:errorcluster)  [unwired: 9 in]
        n194 = call "Read Array.vi"("error in (no error)"=w423, "Controller Array in"=w428) -> ("error out"=w425:errorcluster, "Array"=w427:refnum<class "Generic Plugin.lvclass">[])  [unwired: 7 in, 1 out]
        n195 = for {
          tunnel: w427 -> [w432] mode=indexing
          shift-right: [w431] -> w424
          shift-left: w425 -> [w433]
          n196 = call "Send Stop Message.vi"("error in (no error)"=w433, "Generic Controller in"=w432) -> ("error out"=w431:errorcluster)  [unwired: 8 in, 1 out]
        }
        n197 = call "Ready Status.vi"("error in (no error)"=w424) -> ("error out"=w430:errorcluster)  [unwired: 2 in]
      }
      frame "Load Optimizer" {
        # "Right now we can only load one optimizer at a time, so check if one is already loaded\nin the process cache. If there is one, do not try to load another."
        # "Load a selected process."
        n198 = Unbundle By Name(w447) -> ("Log Directory"=w434:path, "Optimizers.Process Cache"=w438:refnum<class "Controller Array.lvclass">, "Optimizers.Plugins"=w446:T4[])
        n199 = call "Update Status.vi"("error in (no error)"=w444, "Status Bar Text"="Loading Optimizer...") -> ("error out"=w443:errorcluster)  [unwired: 9 in]
        n200 = call "Array Size.vi"("Controller Array in"=w438) -> ("size(s)"=w440:i32)  [unwired: 1 in, 2 out]
        n201 = Less Or Equal To 0?(x=w440) -> (x <= 0?=w439:bool)
        n202 = case shown="True" w439 {
          tunnel: [w449 w461] -> w437
          tunnel: w447 -> [w449 w460]
          tunnel: w446 -> [_ w454]
          tunnel: w443 -> [w448 w459]
          tunnel: w438 -> [_ w457]
          tunnel: [w448 w456] -> w442
          tunnel: w434 -> [_ w455]
          frame False {
          }
          frame True {
            w451 = "Select Optimizer"
            n203 = call "Load Plugin Dialog.vi"("Plugin Selection Ring Text"=w451, "Window Title"=w451, "error in (no error)"=w459, "Plugin List"=w454) -> ("error out"=w458:errorcluster, "cancelled"=w453:bool, "Instance Name"=w450:string, "Plugin Selected"=w452:T4)  [unwired: 4 in]
            n204 = case shown="False" w453 {
              tunnel: [w478 w489] -> w461
              tunnel: w460 -> [w477 w489]
              tunnel: w458 -> [w469 w490]
              tunnel: w457 -> [w476 _]
              tunnel: [w472 w490] -> w456
              tunnel: w455 -> [w465 _]
              tunnel: w452 -> [w470 _]
              tunnel: w450 -> [w464 _]
              frame False {
                n205 = Unbundle By Name(w470) -> ("Controller Type"=w467:T5, "Control Panel Path"=w466:path)
                n206 = call "Initialize Plugin.vi"("Instance Name (blank for default)"=w464, "error in (no error)"=w469, "Log Directory"=w465, "Plugin Path in"=w466, "Plugin Type"=w467) -> ("error out"=w468:errorcluster, "Failed?"=w462:bool, "Generic Controller out"=w463:refnum<class "Generic Plugin.lvclass">)  [unwired: 4 in]
                n207 = case shown="False" w462 {
                  tunnel: w476 -> [w484 w487]
                  tunnel: [w483 w487] -> w475
                  tunnel: [w481 w485] -> w473
                  tunnel: w468 -> [w480 w486]
                  tunnel: w463 -> [w479 _]
                  frame False {
                    n208 = control-ref of="Optimizer Control"() -> (w482:refnum<vi>)
                    n209 = call "Add Optimizer.vi"("Optimizer Control"=w482, "error in (no error)"=w480, "new plugin"=w479, "Plugin Array in"=w484) -> ("error out"=w481:errorcluster, "Plugin Array out"=w483:refnum<class "Controller Array.lvclass">)  [unwired: 6 in]
                  }
                  frame True {
                    # "Clear \"VI already\nclosed\" error that\nsometimes occurs\non abort"
                    n210 = call <vilib>:"Clear Errors.vi"("error in (no error)"=w486, "specific error code to clear (0: all)"=1026) -> ("error out"=w485:errorcluster)  [unwired: 4 in, 1 out]
                  }
                }
                n211 = Bundle By Name(cluster=w477, "Optimizers.Process Cache"=w475) -> (w478:T2)
                n212 = control-ref of="This VI"() -> (w474:refnum<vi>)
                n213 = call "Set Unsaved Changes in Title.vi"("VI in"=w474, "error in (no error)"=w473, "Unsaved changes? (F)"=TRUE) -> ("error out"=w472:errorcluster)  [unwired: 8 in]
              }
              frame True {
              }
            }
          }
        }
        n214 = Unbundle By Name(w437) -> ("Optimizers.Process Cache"=w436:refnum<class "Controller Array.lvclass">)
        n215 = call "Array Size.vi"("Controller Array in"=w436) -> ("size(s)"=→"# of optimizers cached":i32)  [unwired: 1 in, 2 out]
        n216 = call "Ready Status.vi"("error in (no error)"=w442) -> ("error out"=w441:errorcluster)  [unwired: 2 in]
      }
      frame "Stop Optimizer" {
        w512 = "Closing optimizer" ("Status Bar Text")
        # "Remove VI from subpanel"
        # "Stop the current optimizer"
        n217 = Variant To Data(error in=w511, type=w512, Variant=w509) -> (error out=w514:errorcluster)  [unwired: 1 out]
        n218 = call "Update Status.vi"("Status Bar Text"=w512) -> ("error out"=w513:errorcluster)  [unwired: 10 in]
        n219 = Merge Errors(w513, w514) -> (w501:errorcluster)
        n220 = Unbundle By Name(w504) -> ("Optimizers.Process Cache"=w503:refnum<class "Controller Array.lvclass">)
        n221 = call "Index Array.vi"("error in (no error)"=w501, "index"=0, "Controller Array in"=w503) -> ("error out"=w499:errorcluster, "element"=w500:refnum<class "Generic Plugin.lvclass">)  [unwired: 1 out]
        n222 = call "Read Name.vi"("controller in"=w500, "error in (no error)"=w499) -> ("Name"=w497:string, "error out"=w498:errorcluster)  [unwired: 1 out]
        n223 = call "Stop Optimizer VI.vi"("error in (no error)"=w498, "Blocking (T)"=TRUE, "Process Name"=w497, "Data in"=w504) -> ("error out"=w508:errorcluster, "Data out"=w505:T2)  [unwired: 6 in]
        n224 = Unbundle By Name(w505) -> ("Optimizers.Process Cache"=w496:refnum<class "Controller Array.lvclass">, "Message History"=w506:string[][])
        n225 = call "Array Size.vi"("Controller Array in"=w496) -> ("size(s)"=w495:i32)  [unwired: 1 in, 2 out]
        n226 = property on="List of Running Plugins" class="MCListbox (strict)"("ItemNames"=w506) -> ()  [unwired: 2 in, 2 out]
        n227 = local write "# of optimizers cached"(w495) -> ()
        n228 = invoke on="Optimizer Control" class="SubPnl" method="Remove VI"(error in=w508) -> (error out=w493:errorcluster)  [unwired: 2 in, 2 out]
        n229 = control-ref of="This VI"() -> (w494:refnum<vi>)
        n230 = call "Set Unsaved Changes in Title.vi"("VI in"=w494, "error in (no error)"=w493, "Unsaved changes? (F)"=TRUE) -> ("error out"=w492:errorcluster)  [unwired: 8 in]
        n231 = call "Ready Status.vi"("error in (no error)"=w492) -> ("error out"=w510:errorcluster)  [unwired: 2 in]
      }
      frame "New Parameters" {
        w522 = T13 {"Time Stamp"=timestamp(0 s since 1904-01-01), "Names"=[], "Values"=[]}  # New Parameters
        n232 = Unbundle By Name(w530) -> ("Optimizers.First parameters?"=w529:bool, "Parameter to Hardware Map"=w527:refnum<class "Parameter to Hardware Map.lvclass">, "Hardware.Process Cache"=w525:refnum<class "Controller Array.lvclass">)
        n233 = Variant To Data(error in=w528, type=w522, Variant=w523) -> (data=w520:T13, error out=w524:errorcluster)
        n234 = case shown="True" w529 {
          selector: w529 -> [w540 _]
          tunnel: w524 -> [w542 w552]
          tunnel: [w542 w543] -> w518
          tunnel: w527 -> [w541 w554]
          tunnel: w520 -> [_ w553]
          tunnel: w525 -> [_ w550]
          tunnel: [w541 w549] -> w526
          tunnel: [w540 FALSE] -> w521
          frame False {
          }
          frame True {
            n235 = Unbundle By Name(w553) -> ("Names"=w548:string[])
            n236 = for {
              tunnel: w548 -> [w555] mode=indexing
              shift-right: [w557] -> w544
              shift-left: w552 -> [w558]
              shift-right: [w556] -> w551
              shift-left: w554 -> [w559]
              n237 = call "Insert (key-value).vi"("error in (no error)"=w558, "Key"=w555, "Parameter to Hardware Map in"=w559) -> ("error out"=w557:errorcluster, "Parameter to Hardware Map out"=w556:refnum<class "Parameter to Hardware Map.lvclass">)  [unwired: 7 in]
            }
            n238 = call "Assign Parameters to Hardware Dialog.vi"("Hardware Object List"=w550, "Parameter to Hardware Map in"=w551) -> ("Parameter to Hardware Map out"=w549:refnum<class "Parameter to Hardware Map.lvclass">)  [unwired: 9 in]
            n239 = control-ref of="This VI"() -> (w546:refnum<vi>)
            n240 = call "Set Unsaved Changes in Title.vi"("VI in"=w546, "error in (no error)"=w544, "Unsaved changes? (F)"=TRUE) -> ("error out"=w543:errorcluster)  [unwired: 8 in]
          }
        }
        n241 = Bundle By Name(cluster=w530, "Optimizers.First parameters?"=w521, "Parameter to Hardware Map"=w526, "Optimizers.New Parameters"=w520) -> (w516:T2)
        n242 = Unbundle By Name(w516) -> ("Auto Pass Parameters"=w515:bool)
        n243 = case shown="True" w515 {
          tunnel: w519 -> [_ w537]
          tunnel: w518 -> [w535 w539]
          tunnel: [w535 w538] -> w517
          frame False {
            w534 = T14."Enabled" ("Disabled")
            n244 = property on="Accept Suggestions" class="Bool (strict)"("DisabledEnum"=w534, "Value"=FALSE ("Accept Suggestions")) -> ()  [unwired: 2 in, 2 out]
            n245 = property on="Reject Suggestions" class="Bool (strict)"("DisabledEnum"=w534, "Value"=FALSE ("Reject Suggestions")) -> ()  [unwired: 2 in, 2 out]
          }
          frame True {
            n246 = call-poly "Enqueue Message.vi"("error in (no error)"=w539, "Message"="Send Parameters", "Message Queue"=w537) -> ("error out"=w538:errorcluster)  [unwired: 7 in, 1 out]
          }
        }
        n247 = call "Ready Status.vi"("error in (no error)"=w517) -> ("error out"=w531:errorcluster)  [unwired: 2 in]
      }
      frame "Reassign Parameters" {
        # "Reassign parameters to instruments in the Parameter to Hardware Map"
        n248 = Unbundle By Name(w577) -> ("Hardware.Process Cache"=w574:refnum<class "Controller Array.lvclass">, "Optimizers.New Parameters"=w573:T13)
        n249 = call "Update Status.vi"("error in (no error)"=w576, "Status Bar Text"="Reassigning parameters") -> ("error out"=w571:errorcluster)  [unwired: 9 in]
        n250 = Unbundle By Name(w573) -> ("Names"=w563:string[])
        n251 = for {
          tunnel: w563 -> [w579] mode=indexing
          shift-right: [w581] -> w560
          shift-left: w571 -> [w582]
          shift-right: [w580] -> w564
          shift-left: refnum<class "Parameter to Hardware Map.lvclass"> refnum ("Parameter to Hardware Map") -> [w583]
          n252 = call "Insert (key-value).vi"("error in (no error)"=w582, "Key"=w579, "Parameter to Hardware Map in"=w583) -> ("error out"=w581:errorcluster, "Parameter to Hardware Map out"=w580:refnum<class "Parameter to Hardware Map.lvclass">)  [unwired: 7 in]
        }
        n253 = call "Assign Parameters to Hardware Dialog.vi"("Hardware Object List"=w574, "Parameter to Hardware Map in"=w564) -> ("Parameter to Hardware Map out"=w575:refnum<class "Parameter to Hardware Map.lvclass">)  [unwired: 9 in]
        n254 = control-ref of="This VI"() -> (w562:refnum<vi>)
        n255 = call "Set Unsaved Changes in Title.vi"("VI in"=w562, "error in (no error)"=w560, "Unsaved changes? (F)"=TRUE) -> ("error out"=w569:errorcluster)  [unwired: 8 in]
        n256 = Bundle By Name(cluster=w577, "Parameter to Hardware Map"=w575) -> (w566:T2)
        n257 = Unbundle By Name(w566) -> ("Auto Pass Parameters"=w565:bool)
        n258 = case shown="True" w565 {
          tunnel: w567 -> [_ w589]
          tunnel: w569 -> [w587 w591]
          tunnel: [w587 w590] -> w568
          frame False {
            w586 = T14."Enabled" ("Disabled")
            n259 = property on="Accept Suggestions" class="Bool (strict)"("DisabledEnum"=w586, "Value"=FALSE ("Accept Suggestions")) -> ()  [unwired: 2 in, 2 out]
            n260 = property on="Reject Suggestions" class="Bool (strict)"("DisabledEnum"=w586, "Value"=FALSE ("Reject Suggestions")) -> ()  [unwired: 2 in, 2 out]
          }
          frame True {
            n261 = call-poly "Enqueue Message.vi"("error in (no error)"=w591, "Message"="Send Parameters", "Message Queue"=w589) -> ("error out"=w590:errorcluster)  [unwired: 7 in, 1 out]
          }
        }
        n262 = call "Ready Status.vi"("error in (no error)"=w568) -> ("error out"=w578:errorcluster)  [unwired: 2 in]
      }
      frame "Toggle Auto Param Passing" {
        # "Toggles whether parameters are passed automatically or not."
        n263 = Variant To Data(error in=w597, type=FALSE, Variant=w594) -> (data=w592:bool, error out=w595:errorcluster)
        n264 = Bundle By Name(cluster=w598, "Auto Pass Parameters"=w592) -> (w596:T2)
      }
      frame "Submit Goal" {
        # "Submit the goal value(s) to the optimizer(s)"
        n265 = Unbundle By Name(w603) -> ("Optimizers.Process Cache"=w602:refnum<class "Controller Array.lvclass">)
        n266 = call "Array Size.vi"("Controller Array in"=w602) -> ("size(s)"=w600:i32)  [unwired: 1 in, 2 out]
        n267 = Greater Than 0?(x=w600) -> (x > 0?=w601:bool)
        n268 = case shown="True" w601 {
          tunnel: w606 -> [w607 w623]
          tunnel: [w607 w621] -> w605
          tunnel: w604 -> [_ w619]
          tunnel: w602 -> [_ w615]
          frame False {
          }
          frame True {
            w612 = refnum<class "Generic Optimizer.lvclass"> refnum  # Generic Optimizer.lvclass
            n269 = call "Update Status.vi"("error in (no error)"=w623, "Status Bar Text"="Submitting yield") -> ("error out"=w624:errorcluster)  [unwired: 9 in]
            n270 = call "Search Array.vi"("Searchable Property (Name)"=Searchable_Properties."Controller Type", "Search Value"=Controller_Type."Generic Optimizer" ("Controller Type"), "Controller Array in"=w615) -> ("error out"=w610:errorcluster, "Controller found"=w613:refnum<class "Generic Plugin.lvclass">)  [unwired: 1 in, 2 out]
            n271 = Variant To Data(error in=w624, type=0.0, Variant=w619) -> (data=w617:dbl, error out=w620:errorcluster)
            n272 = To More Specific Class(target class=w612, reference=w613, error in=w610) -> (specific class reference=w611:refnum<class "Generic Optimizer.lvclass">, error out=w608:errorcluster)
            n273 = Merge Errors(w608, w620) -> (w609:errorcluster)
            n274 = call-dynamic "Submit Goal.vi"("error in (no error)"=w609, "Goal"=w617, "Generic Optimizer in"=w611) -> ("error out"=w621:errorcluster)  [unwired: 7 in, 1 out]
          }
        }
        n275 = call "Ready Status.vi"("error in (no error)"=w605) -> ("error out"=w599:errorcluster)  [unwired: 2 in]
      }
      frame "Send Parameters" {
        # "Send the optimizer's suggested parameter values to the respective hardware"
        n276 = Unbundle By Name(w627) -> ("Optimizers.First parameters?"=w626:bool)
        n277 = Unbundle By Name(w627) -> ("Parameter to Hardware Map"=w633:refnum<class "Parameter to Hardware Map.lvclass">, "Optimizers.New Parameters"=w630:T13)
        n278 = call "Update Status.vi"("error in (no error)"=w635, "Status Bar Text"="Broadcasting reaction parameters.") -> ("error out"=w632:errorcluster)  [unwired: 9 in]
        n279 = Unbundle By Name(w630) -> ("Names"=w628:string[], "Values"=w629:dbl[])
        n280 = case shown="True" w626 {
          frame False {
            w636 = T14."Disabled and Grayed Out" ("Disabled")
            n281 = property on="Accept Suggestions" class="Bool (strict)"("DisabledEnum"=w636, "Value"=TRUE ("Accept Suggestions")) -> ()  [unwired: 2 in, 2 out]
            n282 = property on="Reject Suggestions" class="Bool (strict)"("DisabledEnum"=w636) -> ()  [unwired: 2 in, 2 out]
          }
          frame True {
            n283 = property on="Accept Suggestions" class="Bool (strict)"("Value"=FALSE ("Accept Suggestions")) -> ()  [unwired: 2 in, 2 out]
          }
        }
        n284 = for {
          tunnel: w633 -> [w646]
          shift-right: [w641] -> w631
          shift-left: w632 -> [w643]
          tunnel: w629 -> [w640] mode=indexing
          tunnel: w628 -> [w639] mode=indexing
          n285 = call "Find (single).vi"("error in (no error)"=w643, "Key"=w639, "Parameter to Hardware Map in"=w646) -> ("error out"=w642:errorcluster, "Key-Value Pair"=w645:T15)  [unwired: 5 in, 2 out]
          n286 = Unbundle By Name(w645) -> ("values"=w644:refnum<class "Generic Plugin.lvclass">[])
          n287 = for {
            tunnel: w644 -> [w650] mode=indexing
            shift-right: [w647] -> w641
            shift-left: w642 -> [w649]
            tunnel: w640 -> [w648]
            n288 = call "Send New Parameter.vi"("error in (no error)"=w649, "New parameter"=w648, "controller in"=w650) -> ("error out"=w647:errorcluster)  [unwired: 7 in, 1 out]
          }
        }
        n289 = call "Ready Status.vi"("error in (no error)"=w631) -> ("error out"=w625:errorcluster)  [unwired: 2 in]
      }
      frame "Reject Parameters" {
        # "Reject the optimizer's suggested values"
        n290 = Unbundle By Name(w655) -> ("Optimizers.First parameters?"=w654:bool)
        n291 = call "Update Status.vi"("error in (no error)"=w657, "Status Bar Text"="Rejecting suggestions; Requesting new ones.") -> ("error out"=w653:errorcluster)  [unwired: 9 in]
        n292 = case shown="False" w654 {
          tunnel: w653 -> [w662 w665]
          tunnel: w651 -> [w659 _]
          tunnel: [w658 w665] -> w652
          frame False {
            w663 = T14."Disabled and Grayed Out" ("Disabled")
            # "Punish optimizer for going\nout of range"
            n293 = call-poly "Enqueue Message.vi"("error in (no error)"=w662, "Message Data"=-1.0, "Message"="Submit Goal", "Message Queue"=w659) -> ("error out"=w658:errorcluster)  [unwired: 6 in, 1 out]
            n294 = property on="Accept Suggestions" class="Bool (strict)"("DisabledEnum"=w663) -> ()  [unwired: 2 in, 2 out]
            n295 = property on="Reject Suggestions" class="Bool (strict)"("DisabledEnum"=w663, "Value"=TRUE ("Reject Suggestions")) -> ()  [unwired: 2 in, 2 out]
          }
          frame True {
            n296 = property on="Reject Suggestions" class="Bool (strict)"("Value"=FALSE ("Reject Suggestions")) -> ()  [unwired: 2 in, 2 out]
          }
        }
      }
      frame "Load Analyzer" {
        # "Right now we can only load one analyzer at a time, so check if one is already loaded\nin the process cache. If there is one, do not try to load another."
        # "Keep the queue reference in memory until the process can\nstart receiving commands"
        # "Stop the current analyzer"
        n297 = Unbundle By Name(w680) -> ("Log Directory"=w667:path, "Analyzers.Process Cache"=w671:refnum<class "Controller Array.lvclass">, "Analyzers.Plugins"=w679:T4[])
        n298 = call "Update Status.vi"("error in (no error)"=w677, "Status Bar Text"="Loading Analyzer...") -> ("error out"=w676:errorcluster)  [unwired: 9 in]
        n299 = call "Array Size.vi"("Controller Array in"=w671) -> ("size(s)"=w673:i32)  [unwired: 1 in, 2 out]
        n300 = Less Or Equal To 0?(x=w673) -> (x <= 0?=w672:bool)
        n301 = case shown="True" w672 {
          tunnel: [w682 w694] -> w670
          tunnel: w680 -> [w682 w693]
          tunnel: w679 -> [_ w686]
          tunnel: w676 -> [w681 w692]
          tunnel: w671 -> [_ w690]
          tunnel: [w681 w689] -> w675
          tunnel: w667 -> [_ w687]
          frame False {
          }
          frame True {
            w684 = "Analyzer Optimizer"
            n302 = call "Load Plugin Dialog.vi"("Plugin Selection Ring Text"=w684, "Window Title"=w684, "error in (no error)"=w692, "Plugin List"=w686) -> ("error out"=w691:errorcluster, "cancelled"=w688:bool, "Instance Name"=w683:string, "Plugin Selected"=w685:T4)  [unwired: 4 in]
            n303 = case shown="False" w688 {
              tunnel: [w711 w722] -> w694
              tunnel: w693 -> [w710 w722]
              tunnel: w691 -> [w702 w723]
              tunnel: w690 -> [w709 _]
              tunnel: [w706 w723] -> w689
              tunnel: w687 -> [w698 _]
              tunnel: w685 -> [w703 _]
              tunnel: w683 -> [w697 _]
              frame False {
                n304 = Unbundle By Name(w703) -> ("Controller Type"=w699:T5, "Control Panel Path"=w700:path)
                n305 = call "Initialize Plugin.vi"("Instance Name (blank for default)"=w697, "error in (no error)"=w702, "Log Directory"=w698, "Plugin Path in"=w700, "Plugin Type"=w699) -> ("error out"=w701:errorcluster, "Failed?"=w695:bool, "Generic Controller out"=w696:refnum<class "Generic Plugin.lvclass">)  [unwired: 4 in]
                n306 = case shown="False" w695 {
                  tunnel: w709 -> [w717 w718]
                  tunnel: [w716 w718] -> w708
                  tunnel: [w715 w719] -> w707
                  tunnel: w701 -> [w713 w720]
                  tunnel: w696 -> [w712 _]
                  frame False {
                    n307 = control-ref of="Analyzer"() -> (w714:refnum<vi>)
                    n308 = call "Add Analyzer.vi"("Analyzer Subpanel"=w714, "error in (no error)"=w713, "new plugin"=w712, "Plugin Array in"=w717) -> ("error out"=w715:errorcluster, "Plugin Array out"=w716:refnum<class "Controller Array.lvclass">)  [unwired: 6 in]
                  }
                  frame True {
                    # "Clear \"VI already\nclosed\" error that\nsometimes occurs\non abort"
                    n309 = call <vilib>:"Clear Errors.vi"("error in (no error)"=w720, "specific error code to clear (0: all)"=1026) -> ("error out"=w719:errorcluster)  [unwired: 4 in, 1 out]
                  }
                }
                n310 = Bundle By Name(cluster=w710, "Analyzers.Process Cache"=w708) -> (w711:T2)
                n311 = control-ref of="This VI"() -> (w705:refnum<vi>)
                n312 = call "Set Unsaved Changes in Title.vi"("VI in"=w705, "error in (no error)"=w707, "Unsaved changes? (F)"=TRUE) -> ("error out"=w706:errorcluster)  [unwired: 8 in]
              }
              frame True {
              }
            }
          }
        }
        n313 = Unbundle By Name(w670) -> ("Analyzers.Process Cache"=w669:refnum<class "Controller Array.lvclass">)
        n314 = call "Array Size.vi"("Controller Array in"=w669) -> ("size(s)"=→"# of analyzers cached":i32)  [unwired: 1 in, 2 out]
        n315 = call "Ready Status.vi"("error in (no error)"=w675) -> ("error out"=w674:errorcluster)  [unwired: 2 in]
      }
      frame "Stop Analyzer" {
        w745 = "Closing analyzer" ("Status Bar Text")
        # "Remove VI from subpanel"
        # "Stop the analyzer and remove it from the subpanel."
        n316 = Variant To Data(error in=w744, type=w745, Variant=w742) -> (error out=w747:errorcluster)  [unwired: 1 out]
        n317 = call "Update Status.vi"("Status Bar Text"=w745) -> ("error out"=w746:errorcluster)  [unwired: 10 in]
        n318 = Merge Errors(w746, w747) -> (w734:errorcluster)
        n319 = Unbundle By Name(w737) -> ("Analyzers.Process Cache"=w736:refnum<class "Controller Array.lvclass">)
        n320 = call "Index Array.vi"("error in (no error)"=w734, "index"=0, "Controller Array in"=w736) -> ("error out"=w732:errorcluster, "element"=w733:refnum<class "Generic Plugin.lvclass">)  [unwired: 1 out]
        n321 = call "Read Name.vi"("controller in"=w733, "error in (no error)"=w732) -> ("Name"=w730:string, "error out"=w731:errorcluster)  [unwired: 1 out]
        n322 = call "Stop Analyzer VI.vi"("error in (no error)"=w731, "Blocking (T)"=TRUE, "Process Name"=w730, "Data in"=w737) -> ("error out"=w741:errorcluster, "Data out"=w738:T2)  [unwired: 6 in]
        n323 = Unbundle By Name(w738) -> ("Analyzers.Process Cache"=w729:refnum<class "Controller Array.lvclass">, "Message History"=w739:string[][])
        n324 = call "Array Size.vi"("Controller Array in"=w729) -> ("size(s)"=w728:i32)  [unwired: 1 in, 2 out]
        n325 = property on="List of Running Plugins" class="MCListbox (strict)"("ItemNames"=w739) -> ()  [unwired: 2 in, 2 out]
        n326 = local write "# of analyzers cached"(w728) -> ()
        n327 = invoke on="Analyzer" class="SubPnl" method="Remove VI"(error in=w741) -> (error out=w725:errorcluster)  [unwired: 2 in, 2 out]
        n328 = control-ref of="This VI"() -> (w727:refnum<vi>)
        n329 = call "Set Unsaved Changes in Title.vi"("VI in"=w727, "error in (no error)"=w725, "Unsaved changes? (F)"=TRUE) -> ("error out"=w724:errorcluster)  [unwired: 8 in]
        n330 = call "Ready Status.vi"("error in (no error)"=w724) -> ("error out"=w743:errorcluster)  [unwired: 2 in]
      }
    }
    n331 = call "Error Handler - Main VI State Machine.vi"("error in (no error)"=w43, "Message Queue"=w41) -> ("dup error in"=w42:errorcluster)  [unwired: 8 in, 1 out]
  }
  n332 = while {
    tunnel: w34 -> [w751]
    tunnel: w33 -> [w749]
    tunnel: [w748] -> w30
    stop <- w750 stop-if-true
    n333 = event shown="[3] Panel Close?" {
      selector: w749 -> [_ _ _ _ _ _ _ _ _ _ _ _ _ _ _ _ _ _ _ _ _ _ _ _ _ _ _ _ _]
      dyn-events: [_ _ _ _ _ _ _ _ _ _ _ _ _ _ _ _ _ _ _ _ _ _ _ _ _ _ _ _ _] -> w748
      timeout: _ -> [_ _ _ _ _ _ _ _ _ _ _ _ _ _ _ _ _ _ _ _ _ _ _ _ _ _ _ _ _]
      tunnel: w751 -> [w754 _ w756 w760 w767 _ _ _ w775 w786 w791 _ w800 w802 w806 w808 w811 w813 w815 w817 _ w825 w828 w831 w836 _ w846 w848 w851]
      tunnel: [_ _ _ _ _ w770 _ _ _ _ _ _ _ _ _ _ _ _ _ _ _ _ _ _ _ _ _ _ _] -> w750
      event "Exit": Value Change {
        # "Begin the exitting process"
        n334 = event-data() -> ()  [unwired: 1 in, 1 out]
        n335 = call-poly "Enqueue Message.vi"("Priority Message? (F)"=TRUE, "Message"="Exitting", "Message Queue"=w754) -> ()  [unwired: 7 in, 2 out]
      }
      event Timeout {
        # "Do nothing on timeout. If no timeout value is given, this should not even be invoked."
        n336 = event-data() -> ()  [unwired: 1 in, 1 out]
      }
      event Application Instance Close {
        n337 = event-data() -> ()  [unwired: 1 in, 1 out]
        n338 = call-poly "Enqueue Message.vi"("Priority Message? (F)"=TRUE, "Message"="Exitting", "Message Queue"=w756) -> ()  [unwired: 7 in, 2 out]
      }
      event Panel Close? {
        n339 = event-data() -> ()  [unwired: 1 in, 1 out]
        n340 = call-poly "Enqueue Message.vi"("Priority Message? (F)"=TRUE, "Message"="Exitting", "Message Queue"=w760) -> ()  [unwired: 7 in, 2 out]
        n341 = event-data("Discard?"=TRUE) -> ()  [unwired: 1 in, 1 out]
      }
      event Key Down {
        w766 = 115  # 's' key
        n342 = event-data() -> ("Char"=w765:i16, "Mods.Menu Key"=w762:bool)  [unwired: 1 in]
        n343 = Equal?(x=w766, y=w765) -> (x = y?=w763:bool)
        n344 = And(x=w763, y=w762) -> (x .and. y?=w764:bool)
        n345 = case shown="True" w764 {
          tunnel: w767 -> [_ w769]
          frame False {
          }
          frame True {
            n346 = call-poly "Enqueue Message.vi"("Message"="Save Experiment", "Message Queue"=w769) -> ()  [unwired: 8 in, 2 out]
          }
        }
      }
      event User Event {
        n347 = event-data() -> ("Stop"=w770:bool)  [unwired: 1 in]
      }
      event User Event {
        n348 = event-data() -> ("Status"=→"Status Bar Text":string)  [unwired: 1 in]
      }
      event User Event {
        n349 = event-data() -> ("VIs"=w773:refnum<class "Controller Array.lvclass">)  [unwired: 1 in]
        n350 = call "Array Size.vi"("Controller Array in"=w773) -> ("size(s)"=→"# of processes cached":i32)  [unwired: 1 in, 2 out]
      }
      event User Event {
        n351 = event-data() -> ("Source"=w781:string, "Destination"=w780:string, "Time Stamp"=w779:timestamp, "Command"=w778:string, "Data"=w777:variant)  [unwired: 1 in]
        n352 = Bundle By Name(cluster=T3 {"Source"="", "Destination"="", "Time Stamp"=timestamp(0 s since 1904-01-01), "Command"="", "Data"=variant} ("Message"), "Source"=w781, "Destination"=w780, "Time Stamp"=w779, "Command"=w778, "Data"=w777) -> (w774:T3)
        n353 = call-poly "Enqueue Message.vi"("Message Data"=w774, "Message"="Cache Message", "Message Queue"=w775) -> ()  [unwired: 7 in, 2 out]
      }
      event User Event {
        # "Stop the selected controller"
        n354 = event-data() -> ("Type"=w783:enum16{"Hardware", "Optimizer", "Analyzer"}, "Name"=w784:string)  [unwired: 1 in]
        n355 = case shown="\"Hardware\", Default" w783 {
          tunnel: ["Stop Hardware" ("Message") "Stop Optimizer" ("Message") "Stop Analyzer" ("Message")] -> w785
          frame "Hardware", Default {
          }
          frame "Optimizer" {
          }
          frame "Analyzer" {
          }
        }
        n356 = call-poly "Enqueue Message.vi"("Message Data"=w784, "Message"=w785, "Message Queue"=w786) -> ()  [unwired: 7 in, 2 out]
      }
      event "Load Control Panel": Value Change {
        # "Send message to load controller"
        n357 = event-data() -> ()  [unwired: 1 in, 1 out]
        n358 = call-poly "Enqueue Message.vi"("Message"="Load Hardware", "Message Queue"=w791) -> ()  [unwired: 8 in, 2 out]
      }
      event "Stop Controller Btn": Value Change {
        # "Stop the selected controller"
        n359 = event-data() -> ()  [unwired: 1 in, 1 out]
        n360 = local read "Select a Plugin"() -> (w792:u16)
        n361 = case shown="Default" w792 {
          selector: w792 -> [_ w794]
          frame 0 {
            # "Do nothing if no plugin is selected"
          }
          frame Default {
            # "Fire a Process Stopped Event, providing\nthe name of the process to be stopped"
            n362 = property on="Select a Plugin" class="Ring (strict)"() -> ("Strings []"=w795:string[])  [unwired: 2 in, 2 out]
            n363 = Index Array(array=w795, index=w794) -> (element=w793:string)
            n364 = Bundle By Name(cluster=T16 {"Name"="", "Type"=enum."Hardware"} ("Process Cluster"), "Name"=w793, "Type"=enum16{"Hardware", "Optimizer"}."Hardware") -> (w796:T16)
            n365 = call "Process Stopped Event.vi"() -> ("Process Stopped"=w799:refnum<user-event>)  [unwired: 11 in]
            n366 = Generate User Event(user event=w799, event data cluster=w796) -> ()  [unwired: 2 in, 2 out]
          }
        }
      }
      event "Start Hardware Run Btn": Value Change {
        n367 = event-data() -> ()  [unwired: 1 in, 4 out]
        n368 = call-poly "Enqueue Message.vi"("Message"="Start Hardware Run", "Message Queue"=w800) -> ()  [unwired: 8 in, 2 out]
      }
      event "Stop Hardware Run Btn": Value Change {
        n369 = event-data() -> ()  [unwired: 1 in, 4 out]
        n370 = call-poly "Enqueue Message.vi"("Message"="Stop Hardware Run", "Message Queue"=w802) -> ()  [unwired: 8 in, 2 out]
      }
      event "Select a Plugin": Value Change {
        n371 = event-data() -> ("NewVal"=w805:u16)  [unwired: 1 in]
        n372 = call-poly "Enqueue Message.vi"("Message Data"=w805, "Message"="New Hardware Selected", "Message Queue"=w806) -> ()  [unwired: 7 in, 2 out]
      }
      event User Event {
        n373 = event-data() -> ("Hardware Index"=w807:i32)  [unwired: 1 in]
        n374 = call-poly "Enqueue Message.vi"("Message Data"=w807, "Message"="New Hardware Selected", "Message Queue"=w808) -> ()  [unwired: 7 in, 2 out]
      }
      event User Event {
        n375 = event-data() -> ()  [unwired: 1 in, 1 out]
        n376 = call-poly "Enqueue Message.vi"("Message"="Refresh Hardware Selector", "Message Queue"=w811) -> ()  [unwired: 8 in, 2 out]
      }
      event "Accept Suggestions": Value Change {
        n377 = event-data() -> ()  [unwired: 1 in, 1 out]
        n378 = call-poly "Enqueue Message.vi"("Message"="Send Parameters", "Message Queue"=w813) -> ()  [unwired: 8 in, 2 out]
      }
      event "Reject Suggestions": Value Change {
        n379 = event-data() -> ()  [unwired: 1 in, 1 out]
        n380 = call-poly "Enqueue Message.vi"("Message"="Reject Parameters", "Message Queue"=w815) -> ()  [unwired: 8 in, 2 out]
      }
      event "Load Optimizer Btn": Value Change {
        n381 = event-data() -> ()  [unwired: 1 in, 1 out]
        n382 = call-poly "Enqueue Message.vi"("Message"="Load Optimizer", "Message Queue"=w817) -> ()  [unwired: 8 in, 2 out]
      }
      event "Stop Optimizer Btn": Value Change {
        # "Fire a Process Stopped Event, leaving\nthe process name blank so it is\ndetermined by the current process"
        n383 = event-data() -> ()  [unwired: 1 in, 1 out]
        n384 = Bundle By Name(cluster=T16 {"Name"="", "Type"=enum."Hardware"} ("Process Cluster"), "Name"="", "Type"=enum16{"Hardware", "Optimizer"}."Optimizer") -> (w821:T16)
        n385 = call "Process Stopped Event.vi"() -> ("Process Stopped"=w822:refnum<user-event>)  [unwired: 11 in]
        n386 = Generate User Event(user event=w822, event data cluster=w821) -> ()  [unwired: 2 in, 2 out]
      }
      event "Auto Param Passing": Value Change {
        n387 = event-data() -> ()  [unwired: 1 in, 1 out]
        n388 = call-poly "Enqueue Message.vi"("Message Data"="Auto Param Passing", "Message"="Toggle Auto Param Passing", "Message Queue"=w825) -> ()  [unwired: 7 in, 2 out]
      }
      event User Event {
        n389 = event-data() -> ("Goal"=w826:dbl)  [unwired: 1 in]
        n390 = call-poly "Enqueue Message.vi"("Message Data"=w826, "Message"="Submit Goal", "Message Queue"=w828) -> ()  [unwired: 7 in, 2 out]
      }
      event User Event {
        w835 = T13 {"Time Stamp"=timestamp(0 s since 1904-01-01), "Names"=[], "Values"=[]}  # New Parameters
        n391 = event-data() -> ("Time Stamp"=w834:timestamp, "Names"=w833:string[], "Values"=w832:dbl[])  [unwired: 1 in]
        n392 = Bundle By Name(cluster=w835, "Time Stamp"=w834, "Names"=w833, "Values"=w832) -> (w830:T13)
        n393 = call-poly "Enqueue Message.vi"("Message Data"=w830, "Message"="New Parameters", "Message Queue"=w831) -> ()  [unwired: 7 in, 2 out]
      }
      event "Load Analyzer Btn": Value Change {
        n394 = event-data() -> ()  [unwired: 1 in, 1 out]
        n395 = call-poly "Enqueue Message.vi"("Message"="Load Analyzer", "Message Queue"=w836) -> ()  [unwired: 8 in, 2 out]
      }
      event "Stop Analyzer Btn": Value Change {
        # "Fire a Process Stopped Event, leaving\nthe process name blank so it is\ndetermined by the current process"
        n396 = event-data() -> ()  [unwired: 1 in, 1 out]
        n397 = Bundle By Name(cluster=T16 {"Name"="", "Type"=enum."Hardware"} ("Process Cluster"), "Name"="", "Type"=enum16{"Hardware", "Optimizer", "Analyzer"}."Analyzer") -> (w842:T16)
        n398 = call "Process Stopped Event.vi"() -> ("Process Stopped"=w843:refnum<user-event>)  [unwired: 11 in]
        n399 = Generate User Event(user event=w843, event data cluster=w842) -> (error out=w838:errorcluster)  [unwired: 2 in, 1 out]
        n400 = call <vilib>:"Simple Error Handler.vi"("error in (no error)"=w838) -> ()  [unwired: 4 in, 5 out]
      }
      event User Event {
        # "Forward the new yield to the optimizer."
        n401 = event-data() -> ("New Yield"=w845:dbl)  [unwired: 1 in]
        n402 = call-poly "Enqueue Message.vi"("Message Data"=w845, "Message"="Submit Goal", "Message Queue"=w846) -> ()  [unwired: 7 in, 2 out]
      }
      event "Reassign Parameters": Value Change {
        # "Forward the new yield to the optimizer."
        n403 = event-data() -> ()  [unwired: 1 in, 1 out]
        n404 = call-poly "Enqueue Message.vi"("Message"="Reassign Parameters", "Message Queue"=w848) -> ()  [unwired: 8 in, 2 out]
      }
      event User Event {
        n405 = event-data() -> ("Path"=w850:path)  [unwired: 1 in]
        n406 = call-poly "Enqueue Message.vi"("Message Data"=w850, "Message"="New Log Path", "Message Queue"=w851) -> ()  [unwired: 7 in, 2 out]
      }
    }
  }
  n407 = disable-structure shown="Enabled" {
    frame Enabled {
    }
    frame Disabled {
    }
  }
  n408 = call "Hardware Subpanels.vi"() -> ()  [unwired: 12 in]
  n409 = vi-ref "Hardware Subpanels.vi"() -> (w39:refnum<vi>)
  n410 = invoke on="Reactor Status Indicators" class="SubPnl" method="Insert VI"("VI Ref"=w39) -> ()  [unwired: 3 in, 4 out]
  n411 = Unregister For Events(event registration refnum=w30) -> (error out=w4:errorcluster)  [unwired: 1 in]
  n412 = Destroy User Event(user event=w8, error in=w4) -> (error out=w29:errorcluster)
  n413 = Destroy User Event(user event=w31, error in=w4) -> (error out=w28:errorcluster)
  n414 = Destroy User Event(user event=w25, error in=w4) -> (error out=w24:errorcluster)
  n415 = Destroy User Event(user event=w32, error in=w4) -> (error out=w20:errorcluster)
  n416 = Destroy User Event(user event=w23, error in=w4) -> (error out=w19:errorcluster)
  n417 = Destroy User Event(user event=w21, error in=w4) -> (error out=w18:errorcluster)
  n418 = Destroy User Event(user event=w22, error in=w4) -> (error out=w16:errorcluster)
  n419 = Destroy User Event(user event=w17, error in=w4) -> (error out=w15:errorcluster)
  n420 = Destroy User Event(user event=w7, error in=w4) -> (error out=w3:errorcluster)
  n421 = Destroy User Event(user event=w6, error in=w4) -> (error out=w2:errorcluster)
  n422 = Destroy User Event(user event=w5, error in=w4) -> (error out=w1:errorcluster)
  n423 = Merge Errors(w29, w28, w24, w20, w19, w18, w16, w15, w3, w2, w1) -> (w27:errorcluster)
  n424 = Merge Errors(w40, w27) -> (w9:errorcluster)
  n425 = disable-structure shown="Default" {
    disable-tunnel: w9 -> [w852 _]
    frame condition #0 (active) {
      n426 = call <vilib>:"Simple Error Handler.vi"("error in (no error)"=w852) -> ()  [unwired: 4 in, 5 out]
    }
    frame condition #1 {
      # "Call Quit LabVIEW if running as a built application."
      n427 = Quit LabVIEW() -> ()  [unwired: 1 in]
    }
  }
